vi "Editor_UI_Main.vi"(11 "manager_daemon":refnum<class "manager_daemon.lvclass">) -> ()   [LabVIEW 2024]
uses:
  <vilib>/sklein/WebView2/Webview2 Control/WebView2 Control.xctl
  CV_Shared_Library/volume.type--enum.ctl
  comic_manager/manager_daemon/manager_daemon.lvclass
  comic_manager/manager_daemon/manager_daemon.lvclass/manager_daemon.ctl
  <vilib>/addons/_JKI Toolkits/State Machine/_JKI_lib_State_Machine.llb/Select State(s)_err__jki_lib_state_machine.vi
  <vilib>/addons/_JKI Toolkits/State Machine/_JKI_lib_State_Machine.llb/Periodic Trigger__ogtk__JKI-SM__jki_lib_state_machine.vi
  <userlib>/_OpenG.lib/file/file.llb/Strip Path Extension - String__ogtk.vi
  <userlib>/_OpenG.lib/file/file.llb/openg_file.lvlib
  <vilib>/addons/_JKI.lib/Serialization/JSON/JKI JSON Serialization.lvlib
  CV_Shared_Library/CV_Shared_Library.lvlib
  <userlib>/_OpenG.lib/array/array.llb/openg_array.lvlib
  comic_manager/manager_daemon/type_defs/VolumeData--cluster.ctl
  comic_manager/manager_daemon/type_defs/IssueData--clustrer.ctl
  <userlib>/_OpenG.lib/array/array.llb/Remove Duplicates from 1D Array (Variant)__ogtk.vi
panel:
  out "target volume":string
  in  "delete issue":bool caption="delete current"
  in  "use rel date":bool caption="delete current"
  out "issue chart":picture
  in  "fix dates":bool caption="delete current"
  out "dup issue dates":string[](array[string])
  out "Unique Dates":bool
  in  "delete volume":bool caption="delete current"
  out "URL":string
  in  "refresh listings":bool
  in  "commit volume type":bool
  in  "volume type":T1 caption="Enum"
  out "last updated":string
  in  "Volume":i32 caption="Numeric"
  in  "issue detail tab control":enum32{"Details", "Cover", "Lists"}(tab)
  out "Rel Date":timestamp format="%<%x>T"
  out "Issue ID":i32 caption="Numeric"
  out "Issue Title":string
  in  "Cover Date":timestamp format="%<%x>T"
  out "Issue Number":string
  in  "issue description":string(xcontrol)
  in  "issue cover":string(xcontrol)
  out "Characters":string[](array[string])
  out "Teams":string[](array[string])
  out "StoryArcs":string[](array[string])
  out "Creators":string[](array[string])
  out "Concepts":string[](array[string])
  in  "sort volume":bool
  in  "to top":bool
  in  "move down":bool
  in  "move up":bool
  in  "issues":i32(listbox)
  out "Start Year":i32 caption="Numeric"
  out "issue count":i32 caption="Numeric"
  out "Sortable Title":string
  in  "Title":string
  in  "volume description":string(xcontrol)
  in  "volumes":i32(listbox)
  in  "Folder":i32(listbox)
  in  "Exit":bool
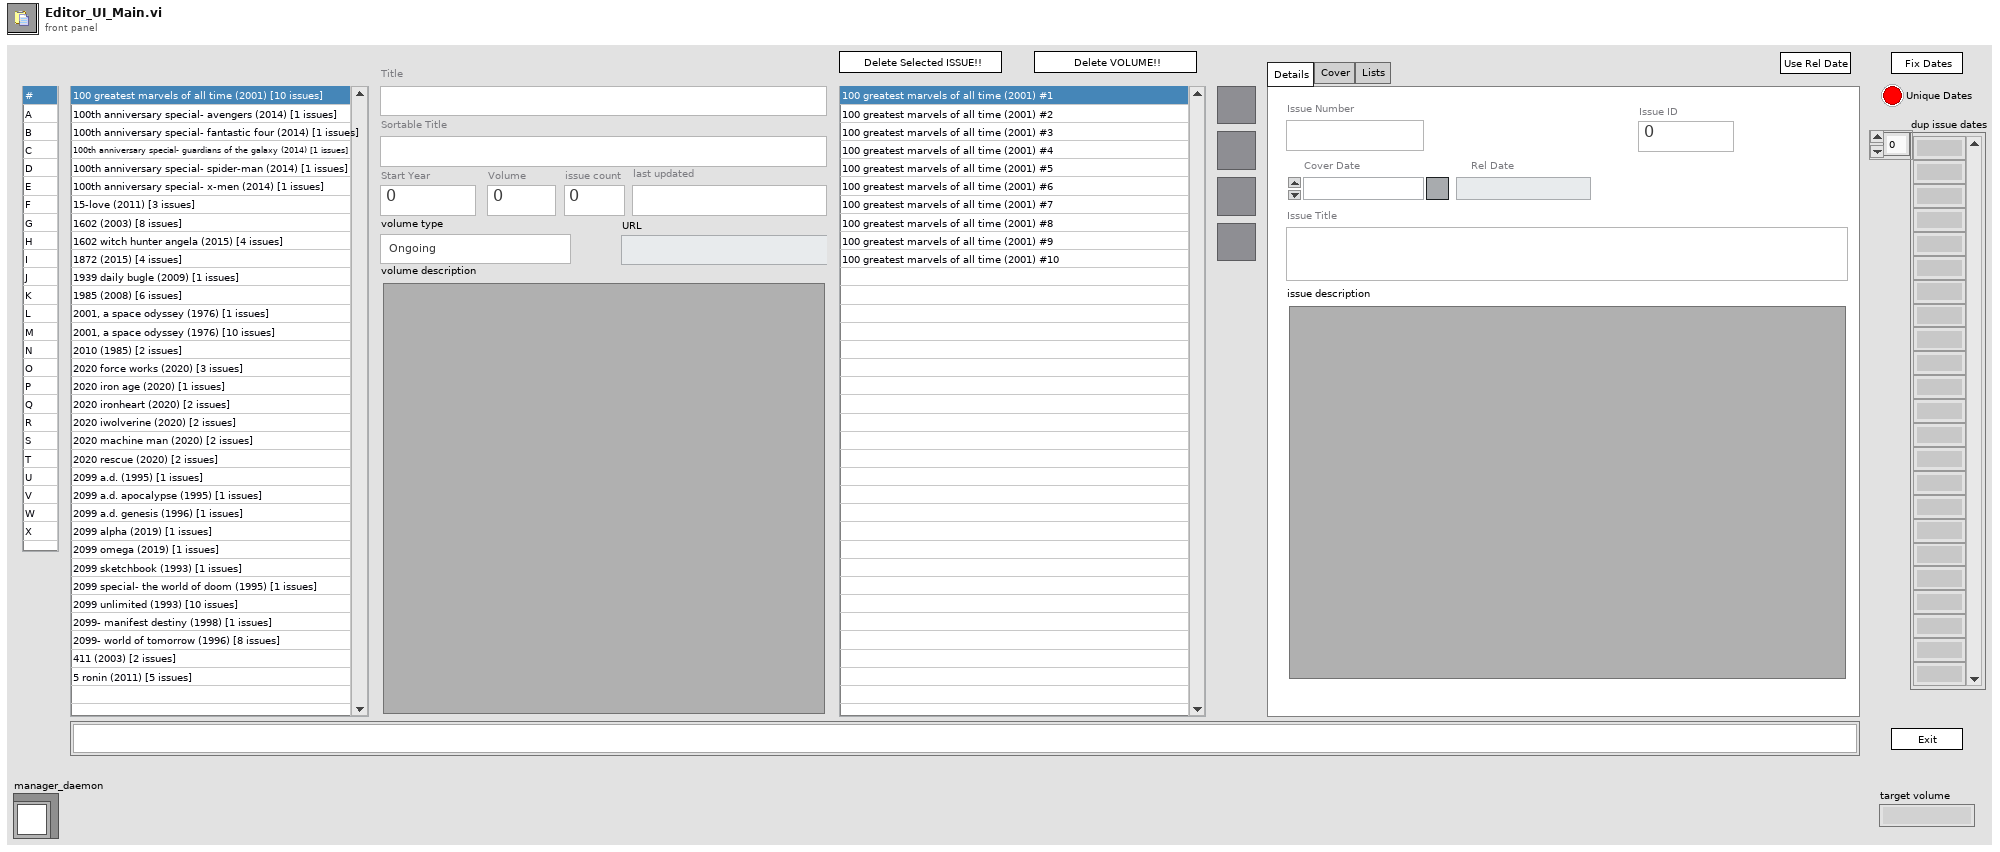
[diagram p1: front panel]
types:
  T1 = typedef "CV_Shared_Library.lvlib/volume.type--enum.ctl" = enum16{"Ongoing", "Limited Series", "Annual", "One Shot", "Reprint/Document", "Star Comics", "Epic Comics"}
  T2 = enum32{"Invalid", "Standard", "Closed", "Hidden", "Minimized", "Maximized"}
  T3 = enum32{"invalid app kind", "Development System", "Run Time System", "Student Edition", "Embedded LabVIEW", "Evaluation", "Custom"}
  T4 = typedef "manager_daemon.lvclass/VolumeData--cluster.ctl" = cluster{"name":string, "sortable_name":string, "aliases":string[], "description":string, "site_detail_url":string, "count_of_issues":i32, "start_year":i32, "publisher_id":i32, "issue_ids":i32[], "date_last_updated":timestamp, "volume":i32, "cv_id":string, "volume type":T1, "source_path":path}
  T5 = typedef "manager_daemon.lvclass/IssueData--clustrer.ctl" = cluster{"cover_date":timestamp, "cv_id":string, "name":string, "sortable_name":string, "issue_number":string, "deck":string, "description":string, "id":i32, "store_date":timestamp, "date_last_updated":timestamp, "site_detail_url":string, "cover_url":string, "source_path":path}
  T6 = cluster{"Core":cluster{"Current VI Reference":refnum<vi>, "Close Panel on Exit?":bool}, "cv_vols":path[], "vol  filter map":map{i32, map{string, i32}}, "current volume map":map{string, i32}, "volume":T4, "issues":T5[], "root paths":cluster{"cv_volumes":path, "cv_issues":path}, "dup issues":i32[], "manager_daemon":refnum<class "manager_daemon.lvclass">, "new volume":string, "Refresh all":bool}
  T7 = cluster{"Current VI Reference":refnum<vi>, "Close Panel on Exit?":bool}
  T8 = typedef "WebView2 Control.xctl/Events.ctl" = cluster{"Navigation Complete Event":refnum<user-event>, "Source Changed Event":refnum<user-event>, "Document Title Changed Event":refnum<user-event>, "Status Bar Text Changed":refnum<user-event>, "Web Message Received":refnum<user-event>, "Window Close Requested":refnum<user-event>, "DOM Loaded":refnum<user-event>, "Navigation Started Event":refnum<user-event>}
  T9 = typedef "CV_RESTful_Lib.lvlib/local_issue--cluster.ctl" = cluster{"cover_date":timestamp, "id":i32, "cv_id":string, "name":string, "sortable_name":string, "issue_number":string, "deck":string, "description":string, "volume":T10, "store_date":timestamp, "date_last_updated":timestamp, "site_detail_url":string, "cover_url":string, "associated_images":T11[], "characters":T10[], "concepts":T10[], "creators":T12[], "storyArcs":T10[], "teams":T10[]}
  T10 = typedef "CV_RESTful_Lib.lvlib/cv_issue.generic_credit--cluster.ctl" = cluster{"id":i32, "name":string}
  T11 = typedef "CV_RESTful_Lib.lvlib/cv_issue.associated_image--cluster.ctl" = cluster{"original_url":string, "id":i32}
  T12 = typedef "CV_RESTful_Lib.lvlib/cv_issue.person_credit--cluster.ctl" = cluster{"id":i32, "name":string, "role":string}
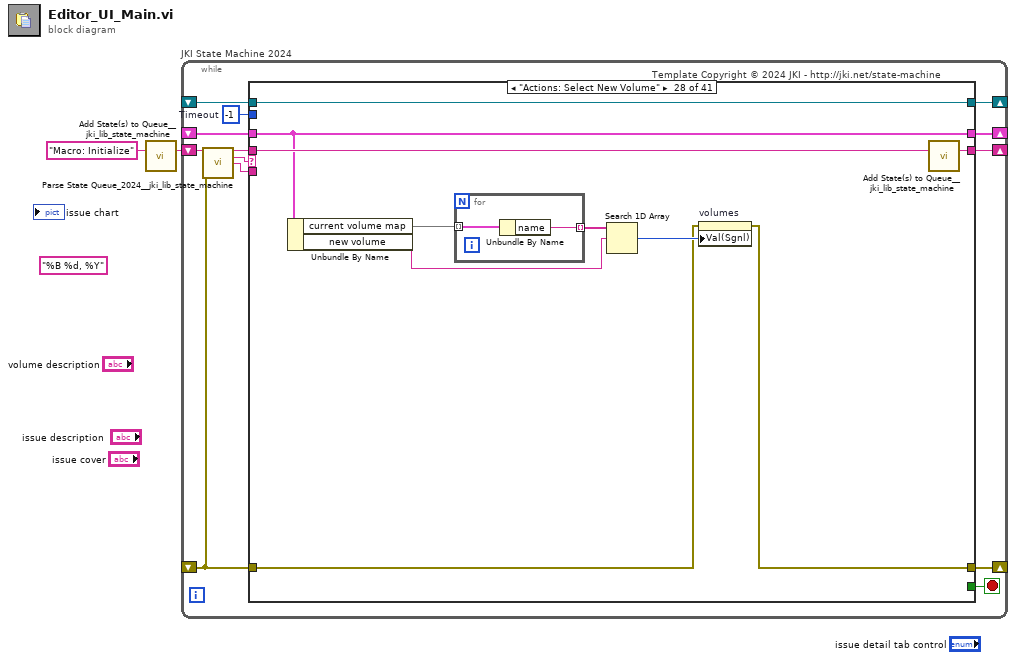
[diagram p0: block diagram]
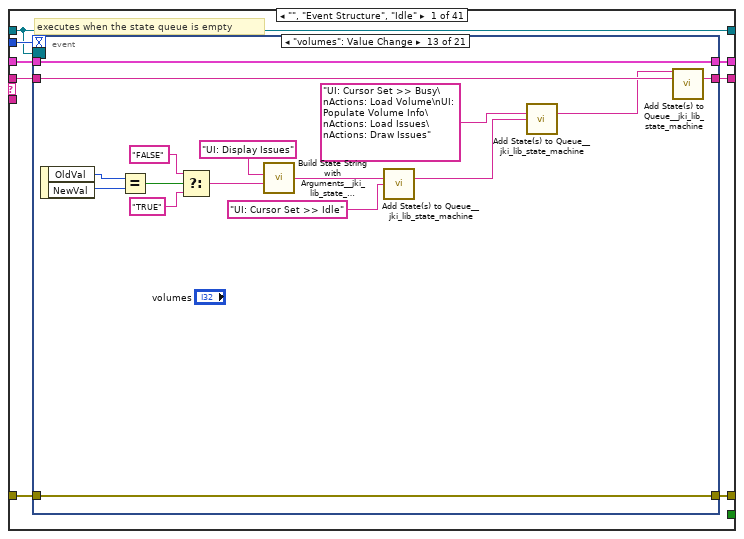
[diagram p2: hidden frame]
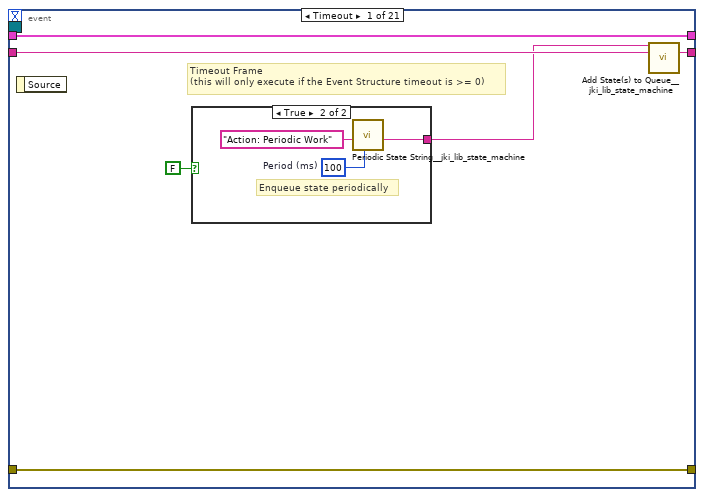
[diagram p3: hidden frame]
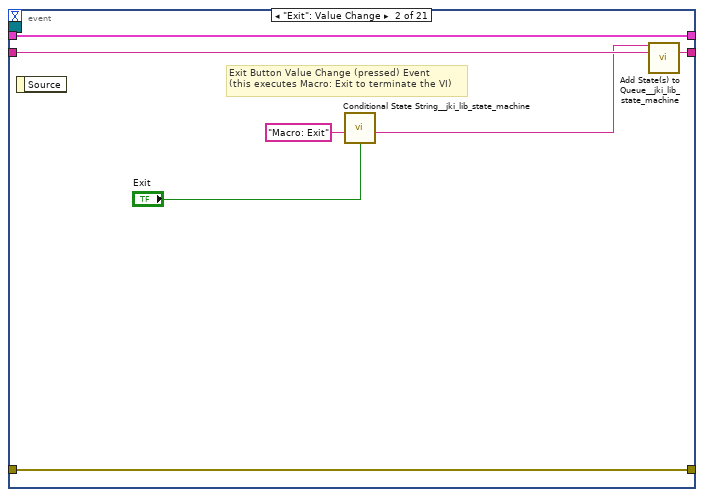
[diagram p5: hidden frame]
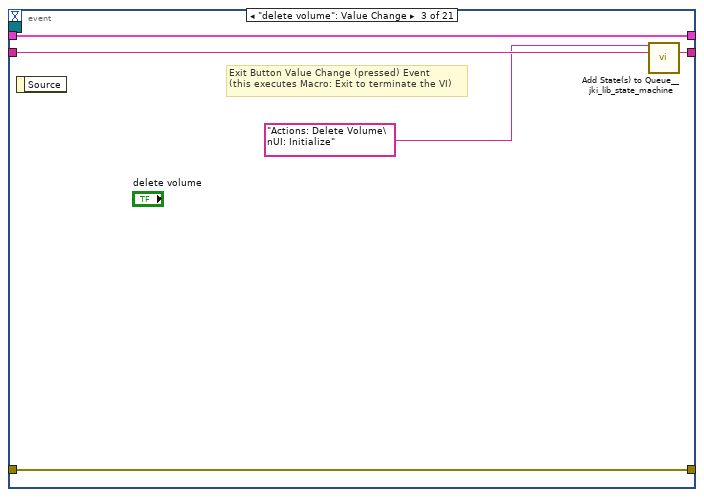
[diagram p6: hidden frame]
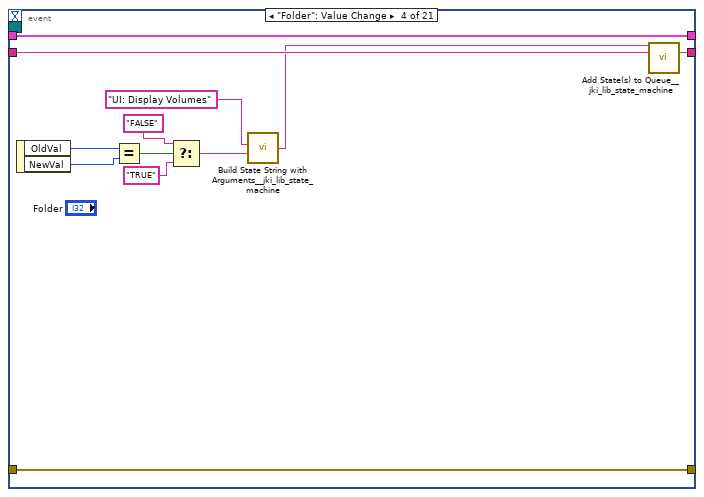
[diagram p7: hidden frame]
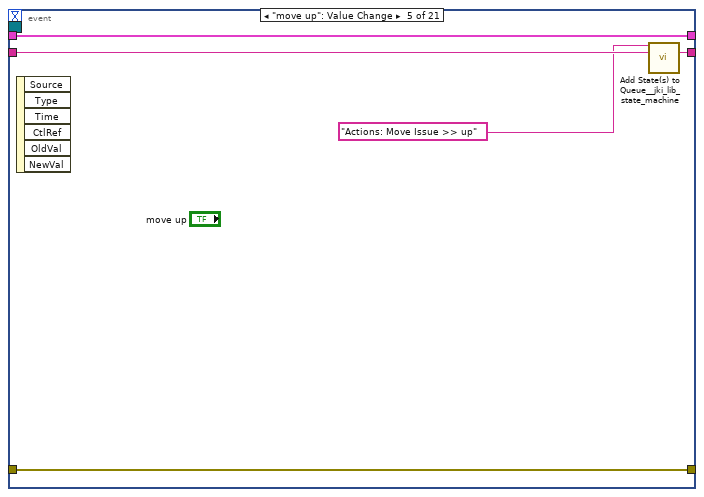
[diagram p8: hidden frame]
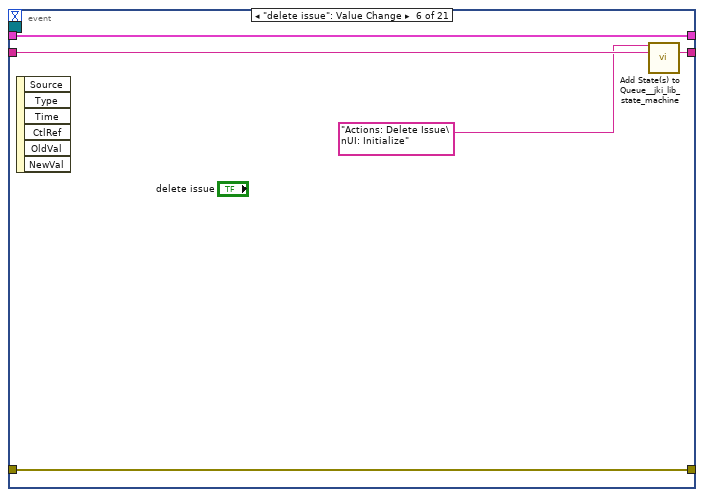
[diagram p9: hidden frame]
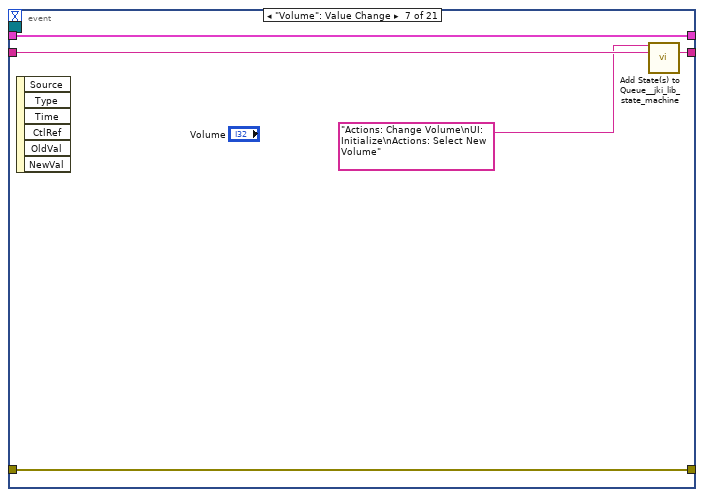
[diagram p10: hidden frame]
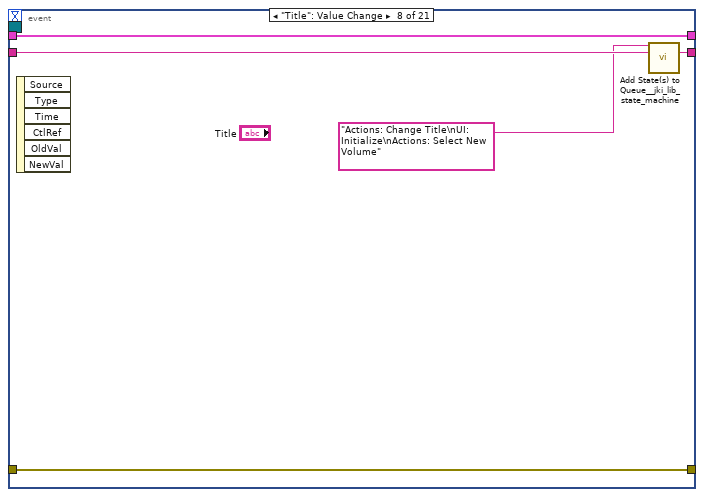
[diagram p11: hidden frame]
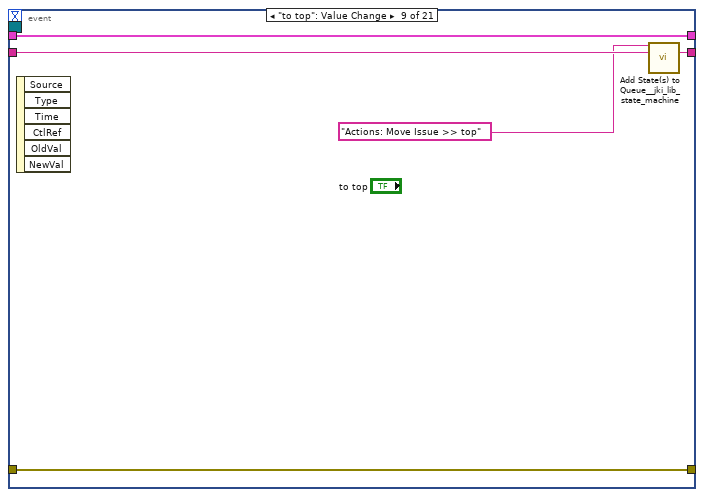
[diagram p12: hidden frame]
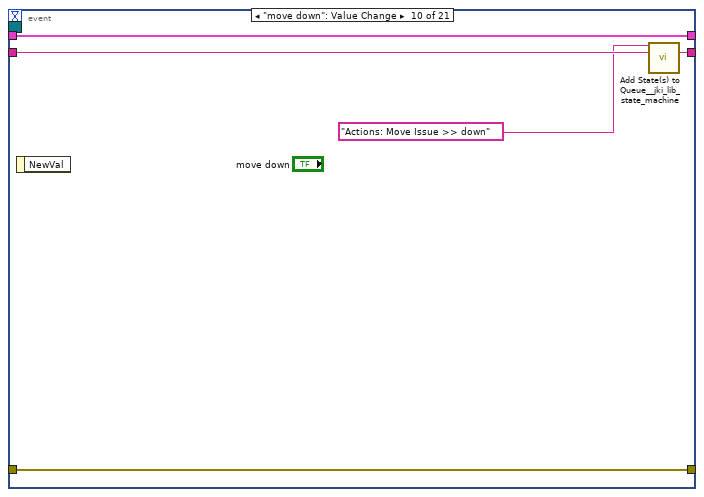
[diagram p13: hidden frame]
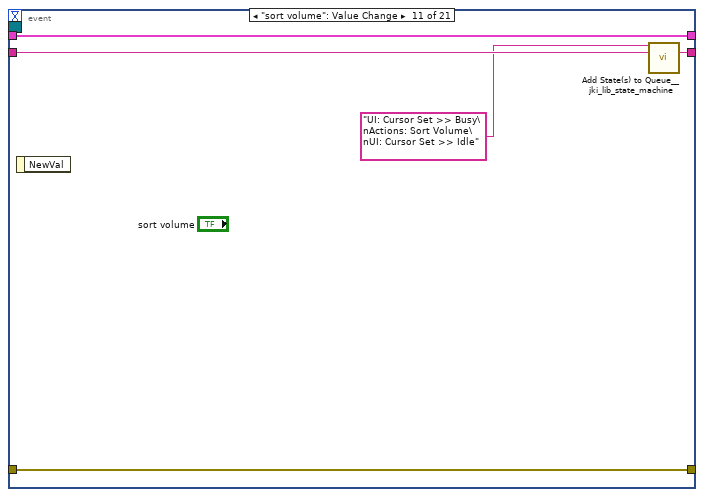
[diagram p14: hidden frame]
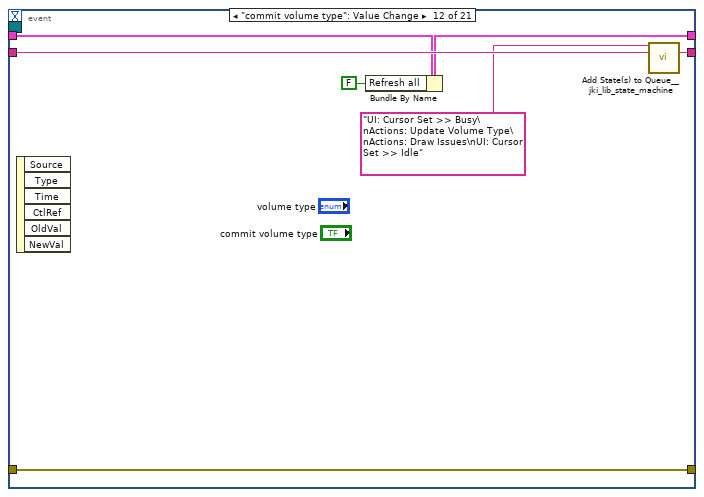
[diagram p15: hidden frame]
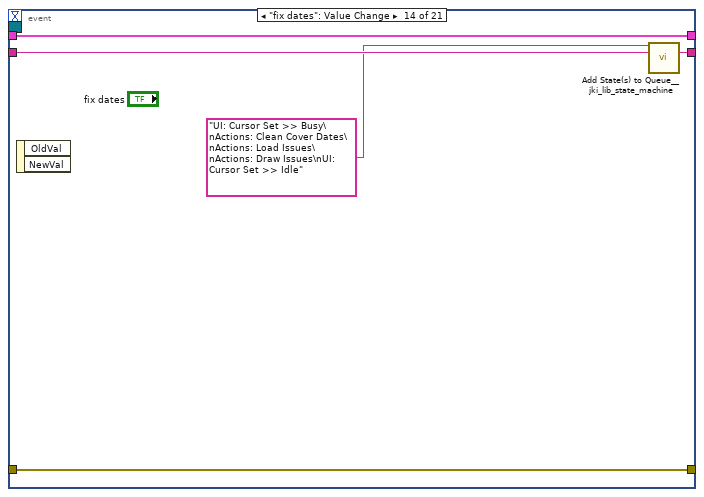
[diagram p16: hidden frame]
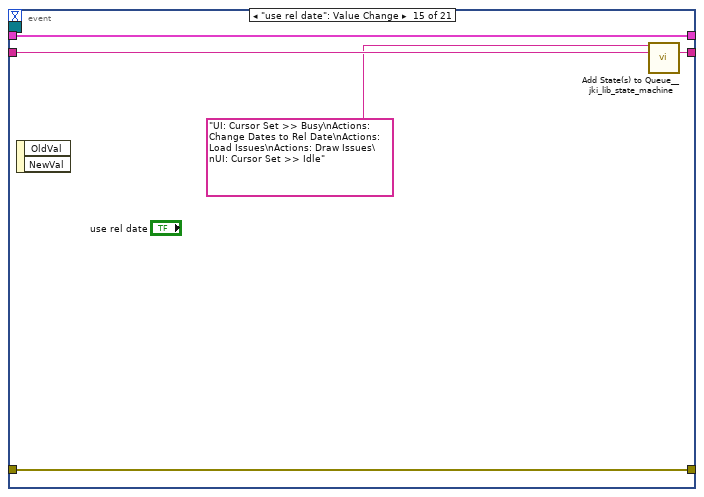
[diagram p17: hidden frame]
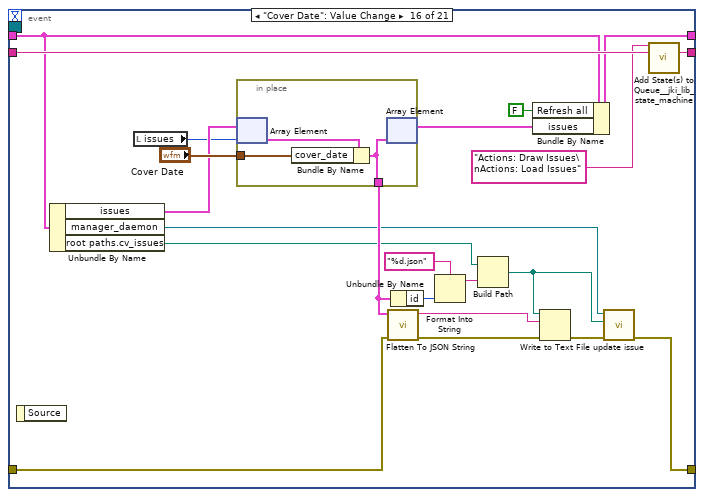
[diagram p18: hidden frame]
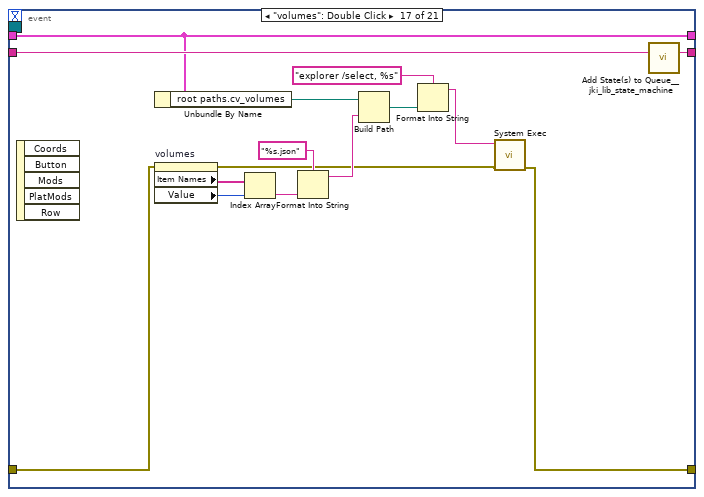
[diagram p19: hidden frame]
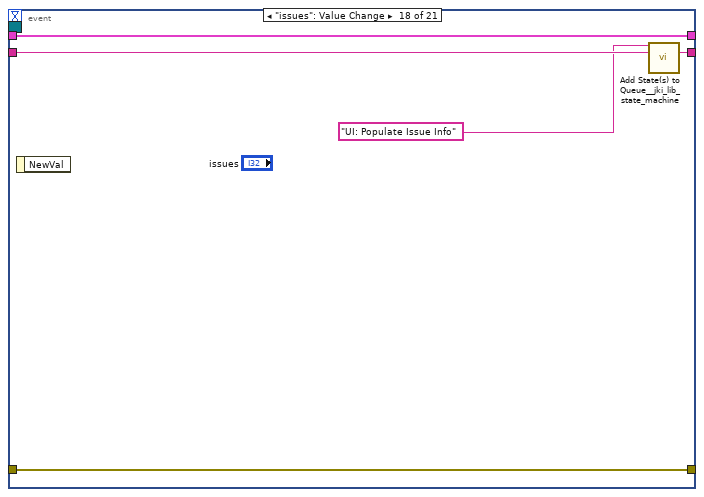
[diagram p20: hidden frame]
diagram:
  (unwired) "%B %d, %Y" ("time format string (%c)")
  n1 = call <vilib>:"Add State(s) to Queue__jki_lib_state_machine.vi"("State(s) in (\"\")"="Macro: Initialize") -> ("States Out"=w2:string)  [unwired: 14 in]
  n2 = while "JKI State Machine 2024" {
    shift-right: [w8] -> _
    shift-left: _ -> [w7]
    shift-right: [w11] -> _
    shift-left: _ -> [w5]
    shift-right: [w10] -> _
    shift-left: w2 -> [w12]
    shift-right: [w4] -> _
    shift-left: _ -> [w3]
    stop <- w9 stop-if-true
    w6 = -1  # Timeout
    # "Template Copyright © 2024 JKI - http://jki.net/state-machine"
    n3 = call <vilib>:"Parse State Queue_2024__jki_lib_state_machine.vi"("State Queue"=w12, "Error In (no error)"=w5) -> ("Remaining States"=w14:string, "Current State"=w15:string, "Arguments"=w13:string)  [unwired: 11 in]
    n4 = case shown="\"Actions: Select New Volume\"" w15 {
      selector: w15 -> [_ _ w217 _ _ _ _ _ _ _ _ _ _ _ _ _ _ _ _ _ _ _ _ _ _ _ _ _ _ _ _ _ _ _ _ _ _ _ _ _ _]
      tunnel: w14 -> [w23 w215 w221 w241 w252 w262 w267 w283 w290 w295 w308 w314 w319 w334 w364 w385 w401 w430 w449 w454 w461 w473 w543 w549 w559 w564 w587 w597 w627 w640 w665 w682 w712 w734 w747 w771 w797 w811 w830 w846 w854]
      tunnel: w13 -> [_ _ _ _ w247 _ _ _ _ _ _ _ _ w322 w356 _ _ _ _ _ w456 w467 _ _ _ _ _ _ _ _ _ _ _ _ _ w753 _ _ _ _ _]
      tunnel: w7 -> [w21 w212 w219 w234 w249 w260 w264 _ w285 w292 w299 w312 w316 w330 w359 w382 w396 w427 w447 w452 w459 w469 w540 w546 w557 w561 w583 w594 w622 w635 w662 w677 w709 w730 w744 w750 w786 w808 w828 w838 w850]
      tunnel: [w20 w213 w223 w238 errorcluster {"status"=FALSE, "code"=0, "source"=""} ("error out") w259 w265 w280 w286 w293 w301 w309 w317 w325 w360 w383 w398 w416 w446 w451 w457 w470 w541 w547 w554 w562 w573 w588 w604 w630 w656 w671 w697 w723 w742 w760 w792 w800 w812 w841 w848] -> w11
      tunnel: w5 -> [w17 w213 w222 w238 w248 w259 w265 w280 w287 w293 w303 w310 w317 w326 w361 w383 w399 w419 w446 w451 w458 w471 w541 w547 w554 w562 w579 w589 w617 w632 w657 w673 w703 w731 w738 w752 w783 w801 w816 w840 w852]
      tunnel: [w22 w214 w220 w240 w251 w261 w266 w282 w289 w294 w307 w313 w318 w333 w363 w384 w400 w429 w448 w453 w460 w472 w542 w548 w558 w563 w586 w596 w626 w639 w664 w681 w711 w733 w746 w770 w796 w810 w830 w845 w854] -> w10
      tunnel: [_ _ _ _ _ TRUE _ _ _ _ _ _ _ _ _ _ _ _ _ _ _ _ _ _ _ _ _ _ _ _ _ _ _ _ _ _ _ _ _ _ _] -> w9
      tunnel: [w19 w212 w219 w239 w249 w260 w264 w281 w285 w292 w299 w312 w316 w329 w359 w382 w396 w427 w447 w452 w459 w469 w540 w546 w557 w561 w584 w594 w624 w633 w662 w676 w709 w730 w737 w749 w785 w807 w827 w842 w853] -> w8
      tunnel: w6 -> [w18 _ _ _ _ _ _ _ _ _ _ _ _ _ _ _ _ _ _ _ _ _ _ _ _ _ _ _ _ _ _ _ _ _ _ _ _ _ _ _ _]
      tunnel: [w16 w211 w216 w228 w242 w257 w263 w277 w284 w291 w304 w311 w315 w324 w362 w381 w397 w428 w444 w450 w455 w466 w539 w544 w550 w560 w585 w595 w625 w638 w663 w680 w710 w732 w745 w769 w795 w809 w829 w839 w851] -> w4
      tunnel: w3 -> [w16 w211 w216 w228 w242 w257 w263 w277 w284 w291 _ w311 w315 w324 w362 w381 w397 w428 w444 w450 w455 w466 w539 w544 w550 w560 w585 w595 w625 w638 w663 w680 w710 w732 w745 w769 w795 w809 w829 w839 w851]
      frame "", "Event Structure", "Idle" {
        # "executes when the state queue is empty"
        n5 = event shown="[12] \"volumes\": Value Change" {
          selector: w16 -> [_ _ _ _ _ _ _ _ _ _ _ _ _ _ _ _ _ _ _ _ _]
          dyn-events: _ -> [_ _ _ _ _ _ _ _ _ _ _ _ _ _ _ _ _ _ _ _ _]
          timeout: w18 -> [_ _ _ _ _ _ _ _ _ _ _ _ _ _ _ _ _ _ _ _ _]
          tunnel: w23 -> [w29 w39 w44 w56 w61 w66 w71 w76 w81 w86 w91 w98 w114 w119 w124 w146 w164 w169 w180 w192 w210]
          tunnel: [w28 w38 w43 w55 w60 w65 w70 w75 w80 w85 w90 w97 w113 w118 w123 w145 w163 w168 w179 w192 w209] -> w22
          tunnel: w21 -> [w26 w36 w41 w53 w58 w63 w68 w73 w78 w83 w88 w94 w111 w116 w121 w141 w158 w166 w174 w193 w207]
          tunnel: [w27 w37 w42 w54 w59 w64 w69 w74 w79 w84 w89 w96 w112 w117 w122 w129 w150 w167 w178 w188 w208] -> w20
          tunnel: w17 -> [w27 w37 w42 w54 w59 w64 w69 w74 w79 w84 w89 w96 w112 w117 w122 w138 w155 w167 w178 w203 w208]
          tunnel: [w26 w36 w41 w53 w58 w63 w68 w73 w78 w83 w88 w93 w111 w116 w121 w139 w158 w166 w170 w193 w207] -> w19
          event Timeout {
            # "Timeout Frame\n(this will only execute if the Event Structure timeout is >= 0)"
            n6 = event-data() -> ()  [unwired: 1 in, 1 out]
            n7 = case shown="True" FALSE {
              tunnel: [_ w32] -> w25
              frame False {
              }
              frame True {
                w30 = u32 100  # Period (ms)
                # "Enqueue state periodically"
                n8 = call <vilib>:"Periodic State String__jki_lib_state_machine.vi"("Period (ms)"=w30, "State"="Action: Periodic Work") -> ("State Out"=w32:string)  [unwired: 9 in]
              }
            }
            n9 = call <vilib>:"Add State(s) to Queue__jki_lib_state_machine.vi"("State(s) in Front (\"\")"=w25, "State(s) in (\"\")"=w29) -> ("States Out"=w28:string)  [unwired: 13 in]
          }
          event "Exit": Value Change {
            # "Exit Button Value Change (pressed) Event\n(this executes Macro: Exit to terminate the VI)"
            n10 = event-data() -> ()  [unwired: 1 in, 1 out]
            n11 = call <vilib>:"Conditional State String__jki_lib_state_machine.vi"("Do State(s)?"="Exit", "State"="Macro: Exit") -> ("State Out"=w33:string)  [unwired: 7 in]
            n12 = call <vilib>:"Add State(s) to Queue__jki_lib_state_machine.vi"("State(s) in Front (\"\")"=w33, "State(s) in (\"\")"=w39) -> ("States Out"=w38:string)  [unwired: 13 in]
          }
          event "delete volume": Value Change {
            # "Exit Button Value Change (pressed) Event\n(this executes Macro: Exit to terminate the VI)"
            n13 = event-data() -> ()  [unwired: 1 in, 1 out]
            n14 = call <vilib>:"Add State(s) to Queue__jki_lib_state_machine.vi"("State(s) in Front (\"\")"="Actions: Delete Volume\nUI: Initialize", "State(s) in (\"\")"=w44) -> ("States Out"=w43:string)  [unwired: 13 in]
          }
          event "Folder": Value Change {
            n15 = event-data() -> ("OldVal"=w52:i32, "NewVal"=w51:i32)  [unwired: 1 in]
            n16 = Equal?(x=w52, y=w51) -> (x = y?=w50:bool)
            n17 = Select(t="FALSE", s=w50, f="TRUE") -> (s? t:f=w46:string)
            n18 = call <vilib>:"Build State String with Arguments__jki_lib_state_machine.vi"("Arguments (\"\")"=w46, "State"="UI: Display Volumes") -> ("State with Arguments"=w45:string)  [unwired: 4 in]
            n19 = call <vilib>:"Add State(s) to Queue__jki_lib_state_machine.vi"("State(s) in Front (\"\")"=w45, "State(s) in (\"\")"=w56) -> ("States Out"=w55:string)  [unwired: 13 in]
          }
          event "move up": Value Change {
            n20 = event-data() -> ()  [unwired: 1 in, 6 out]
            n21 = call <vilib>:"Add State(s) to Queue__jki_lib_state_machine.vi"("State(s) in Front (\"\")"="Actions: Move Issue >> up", "State(s) in (\"\")"=w61) -> ("States Out"=w60:string)  [unwired: 13 in]
          }
          event "delete issue": Value Change {
            n22 = event-data() -> ()  [unwired: 1 in, 6 out]
            n23 = call <vilib>:"Add State(s) to Queue__jki_lib_state_machine.vi"("State(s) in Front (\"\")"="Actions: Delete Issue\nUI: Initialize", "State(s) in (\"\")"=w66) -> ("States Out"=w65:string)  [unwired: 13 in]
          }
          event "Volume": Value Change {
            n24 = event-data() -> ()  [unwired: 1 in, 6 out]
            n25 = call <vilib>:"Add State(s) to Queue__jki_lib_state_machine.vi"("State(s) in Front (\"\")"="Actions: Change Volume\nUI: Initialize\nActions: Select New Volume", "State(s) in (\"\")"=w71) -> ("States Out"=w70:string)  [unwired: 13 in]
          }
          event "Title": Value Change {
            n26 = event-data() -> ()  [unwired: 1 in, 6 out]
            n27 = call <vilib>:"Add State(s) to Queue__jki_lib_state_machine.vi"("State(s) in Front (\"\")"="Actions: Change Title\nUI: Initialize\nActions: Select New Volume", "State(s) in (\"\")"=w76) -> ("States Out"=w75:string)  [unwired: 13 in]
          }
          event "to top": Value Change {
            n28 = event-data() -> ()  [unwired: 1 in, 6 out]
            n29 = call <vilib>:"Add State(s) to Queue__jki_lib_state_machine.vi"("State(s) in Front (\"\")"="Actions: Move Issue >> top", "State(s) in (\"\")"=w81) -> ("States Out"=w80:string)  [unwired: 13 in]
          }
          event "move down": Value Change {
            n30 = event-data() -> ()  [unwired: 1 in, 1 out]
            n31 = call <vilib>:"Add State(s) to Queue__jki_lib_state_machine.vi"("State(s) in Front (\"\")"="Actions: Move Issue >> down", "State(s) in (\"\")"=w86) -> ("States Out"=w85:string)  [unwired: 13 in]
          }
          event "sort volume": Value Change {
            n32 = event-data() -> ()  [unwired: 1 in, 1 out]
            n33 = call <vilib>:"Add State(s) to Queue__jki_lib_state_machine.vi"("State(s) in Front (\"\")"="UI: Cursor Set >> Busy\nActions: Sort Volume\nUI: Cursor Set >> Idle", "State(s) in (\"\")"=w91) -> ("States Out"=w90:string)  [unwired: 13 in]
          }
          event "commit volume type": Value Change {
            n34 = event-data() -> ()  [unwired: 1 in, 6 out]
            n35 = Bundle By Name(cluster=w94, "Refresh all"=FALSE) -> (w93:T6)
            n36 = call <vilib>:"Add State(s) to Queue__jki_lib_state_machine.vi"("State(s) in Front (\"\")"="UI: Cursor Set >> Busy\nActions: Update Volume Type\nActions: Draw Issues\nUI: Cursor Set >> Idle", "State(s) in (\"\")"=w98) -> ("States Out"=w97:string)  [unwired: 13 in]
          }
          event "volumes": Value Change {
            n37 = event-data() -> ("OldVal"=w109:i32, "NewVal"=w110:i32)  [unwired: 1 in]
            n38 = Equal?(x=w109, y=w110) -> (x = y?=w106:bool)
            n39 = Select(t="FALSE", s=w106, f="TRUE") -> (s? t:f=w104:string)
            n40 = call <vilib>:"Build State String with Arguments__jki_lib_state_machine.vi"("Arguments (\"\")"=w104, "State"="UI: Display Issues") -> ("State with Arguments"=w101:string)  [unwired: 4 in]
            n41 = call <vilib>:"Add State(s) to Queue__jki_lib_state_machine.vi"("State(s) in (\"\")"=w101, "State(s) at Back (\"\")"="UI: Cursor Set >> Idle" ("State(s) at Back (\"\")")) -> ("States Out"=w100:string)  [unwired: 13 in]
            n42 = call <vilib>:"Add State(s) to Queue__jki_lib_state_machine.vi"("State(s) in (\"\")"="UI: Cursor Set >> Busy\nActions: Load Volume\nUI: Populate Volume Info\nActions: Load Issues\nActions: Draw Issues", "State(s) at Back (\"\")"=w100) -> ("States Out"=w107:string)  [unwired: 13 in]
            n43 = call <vilib>:"Add State(s) to Queue__jki_lib_state_machine.vi"("State(s) in Front (\"\")"=w107, "State(s) in (\"\")"=w114) -> ("States Out"=w113:string)  [unwired: 13 in]
          }
          event "fix dates": Value Change {
            n44 = event-data() -> ()  [unwired: 1 in, 2 out]
            n45 = call <vilib>:"Add State(s) to Queue__jki_lib_state_machine.vi"("State(s) in Front (\"\")"="UI: Cursor Set >> Busy\nActions: Clean Cover Dates\nActions: Load Issues\nActions: Draw Issues\nUI: Cursor Set >> Idle", "State(s) in (\"\")"=w119) -> ("States Out"=w118:string)  [unwired: 13 in]
          }
          event "use rel date": Value Change {
            n46 = event-data() -> ()  [unwired: 1 in, 2 out]
            n47 = call <vilib>:"Add State(s) to Queue__jki_lib_state_machine.vi"("State(s) in Front (\"\")"="UI: Cursor Set >> Busy\nActions: Change Dates to Rel Date\nActions: Load Issues\nActions: Draw Issues\nUI: Cursor Set >> Idle", "State(s) in (\"\")"=w124) -> ("States Out"=w123:string)  [unwired: 13 in]
          }
          event "Cover Date": Value Change {
            n48 = event-data() -> ()  [unwired: 1 in, 1 out]
            n49 = Unbundle By Name(w141) -> ("issues"=w143:T5[], "manager_daemon"=w127:refnum<class "manager_daemon.lvclass">, "root paths.cv_issues"=w128:path)
            n50 = local read "issues"() -> (w142:i32)
            n51 = in-place {
              in-place-border: "Cover Date" -> [w148]
              in-place-border: [w147] -> w137
              n52 = in-place-array #1(w143, w142) -> (w149:T5)
              n53 = Bundle By Name(cluster=w149, "cover_date"=w148) -> (w147:T5)
              n54 = in-place-array #1(w147) -> (w140:T5[])  [unwired: 1 out]
            }
            n55 = call <vilib>:"Flatten To JSON String.vi"("error in"=w138, "Variant"=w137) -> ("error out"=w132:errorcluster, "JSON String"=w133:string)  [unwired: 8 in]
            n56 = Unbundle By Name(w137) -> ("id"=w136:i32)
            n57 = Format Into String(format string="%d.json", w136) -> (resulting string=w134:string)  [unwired: 2 in, 1 out]
            n58 = Build Path(base path=w128, name or relative path=w134) -> (appended path=w126:path)
            n59 = Bundle By Name(cluster=w141, "Refresh all"=FALSE, "issues"=w140) -> (w139:T6)
            n60 = Write to Text File(file (use dialog)=w126, text=w133, error in=w132) -> (error out=w130:errorcluster)  [unwired: 1 in, 2 out]
            n61 = call "update issue.vi"("error in (no error)"=w130, "Issue Path"=w126, "manager_daemon in"=w127) -> ("error out"=w129:errorcluster)  [unwired: 7 in, 1 out]
            n62 = call <vilib>:"Add State(s) to Queue__jki_lib_state_machine.vi"("State(s) in Front (\"\")"="Actions: Draw Issues\nActions: Load Issues" ("State(s) in Front (\"\")"), "State(s) in (\"\")"=w146) -> ("States Out"=w145:string)  [unwired: 13 in]
          }
          event "volumes": Double Click {
            n63 = event-data() -> ()  [unwired: 1 in, 5 out]
            n64 = Unbundle By Name(w158) -> ("root paths.cv_volumes"=w157:path)
            n65 = property on="volumes" class="LstBox (strict)"(error in=w155) -> (error out=w151:errorcluster, "Item Names"=w161:string[], "Value"=w162:i32)  [unwired: 1 in, 1 out]
            n66 = Index Array(array=w161, index=w162) -> (element=w159:string)
            n67 = Format Into String(format string="%s.json", w159) -> (resulting string=w156:string)  [unwired: 2 in, 1 out]
            n68 = Build Path(base path=w157, name or relative path=w156) -> (appended path=w153:path)
            n69 = Format Into String(format string="explorer /select, %s", w153) -> (resulting string=w152:string)  [unwired: 2 in, 1 out]
            n70 = call <vilib>:"System Exec.vi"("error in (no error)"=w151, "command line"=w152) -> ("error out"=w150:errorcluster)  [unwired: 6 in, 3 out]
            n71 = call <vilib>:"Add State(s) to Queue__jki_lib_state_machine.vi"("State(s) in (\"\")"=w164) -> ("States Out"=w163:string)  [unwired: 14 in]
          }
          event "issues": Value Change {
            n72 = event-data() -> ()  [unwired: 1 in, 1 out]
            n73 = call <vilib>:"Add State(s) to Queue__jki_lib_state_machine.vi"("State(s) in Front (\"\")"="UI: Populate Issue Info", "State(s) in (\"\")"=w169) -> ("States Out"=w168:string)  [unwired: 13 in]
          }
          event "refresh listings": Value Change; User Event {
            (unwired) "UI: Initialize\nActions: Select New Volume"
            n74 = event-data() -> ()  [unwired: 1 in, 3 out]
            n75 = property on="volumes" class="LstBox (strict)"() -> ("Item Names"=w176:string[], "Value"=w175:i32)  [unwired: 2 in, 2 out]
            n76 = Unbundle By Name(w174) -> ("Refresh all"=w173:bool)
            n77 = case shown="True" w173 {
              tunnel: [_ "UI: Initialize"] -> w177
              tunnel: w176 -> [_ w186]
              tunnel: w175 -> [_ w185]
              tunnel: w174 -> [w181 w184]
              tunnel: [w181 w182] -> w172
              frame False {
              }
              frame True {
                n78 = Index Array(array=w186, index=w185) -> (element=w183:string)
                n79 = Bundle By Name(cluster=w184, "new volume"=w183) -> (w182:T6)
              }
            }
            n80 = Bundle By Name(cluster=w172, "Refresh all"=TRUE) -> (w170:T6)
            n81 = call <vilib>:"Add State(s) to Queue__jki_lib_state_machine.vi"("State(s) in Front (\"\")"=w177, "State(s) in (\"\")"=w180) -> ("States Out"=w179:string)  [unwired: 13 in]
          }
          event User Event {
            n82 = event-data() -> ("display volume"=w194:string)  [unwired: 1 in]
            "target volume" <- w194
            n83 = property on="Folder" class="LstBox (strict)"(error in=w203) -> (error out=w195:errorcluster, "Item Names"=w202:string[])  [unwired: 1 in, 1 out]
            n84 = String Subset(string=w194, length (rest)=1 ("length (rest)")) -> (substring=w200:string)  [unwired: 1 in]
            n85 = To Lower Case(string=w202) -> (all lower case string=w201:string[])
            n86 = Search 1D Array(1D array=w201, element=w200) -> (index of element=w198:i32)  [unwired: 1 in]
            n87 = Less Than 0?(x=w198) -> (x < 0?=w199:bool)
            n88 = Select(t=0, s=w199, f=w198) -> (s? t:f=w196:i32)
            n89 = property on="Folder" class="LstBox (strict)"(error in=w195, "Val(Sgnl)"=w196) -> (error out=w189:errorcluster)  [unwired: 1 in, 1 out]
            n90 = control-ref of="This VI"() -> (w191:refnum<vi>)
            n91 = property class="VI"(reference=w191, error in=w189, "Front Panel.IsFrontmost"=TRUE ("Front Panel Window:Is Frontmost")) -> (error out=w188:errorcluster)  [unwired: 1 out]
          }
          event Panel Close? {
            # "Discard the event because we'll close the front panel ourselves in Macro: Exit"
            # "Close Panel button (pressed) Event\n(this executes Macro: Exit to terminate the VI)"
            n92 = event-data() -> ()  [unwired: 1 in, 1 out]
            n93 = event-data("Discard?"=TRUE) -> ()  [unwired: 1 in, 1 out]
            n94 = call <vilib>:"Add State(s) to Queue__jki_lib_state_machine.vi"("State(s) in Front (\"\")"="Macro: Exit", "State(s) in (\"\")"=w210) -> ("States Out"=w209:string)  [unwired: 13 in]
          }
        }
      }
      frame "---------- Core ----------" {
        # "Do not put any code in this frame.\n(it is a separator no-op)"
        n95 = call <vilib>:"Add State(s) to Queue__jki_lib_state_machine.vi"("State(s) in (\"\")"=w215) -> ("States Out"=w214:string)  [unwired: 14 in]
      }
      frame Default {
        w226 = 42 items=["No error", "Argument error", "Memory is full", "Out of zone", "End of file", "File already open", "Generic file I/O error", "File not found", "File permission error", "Disk is full", "Duplicate path", "Too many files open", "System feature not enabled", "Resource file not found", "Cannot add resource", "Resource not found", "Image not found", "Image memory error", "Pen does not exist", "Config type invalid", "Config token not found", "Config parse error", "Config memory error", "Bad external code format", "Bad external code offset", "External code not present", "Null window", "Destroy window error", "Null menu", "Print aborted", "Bad print record", "Print driver error", "Windows error during printing", "Memory error during printing", "Print dialog error", "Generic print error", "Invalid device refnum", "Device not found", "Device parameter error", "Device unit error", "Cannot open device", "Device call aborted", "Generic error", "Cancelled by user", "Object ID too low", "Object ID too high", "Object not in heap", "Unknown heap", "Unknown object (invalid DefProc)", "Unknown object (DefProc not in table)", "Message out of range", "Invalid (null) method", "Unknown message", "Manager call not supported", "Bad address", "Network operation in progress", "Network operation timed out", "Connection is busy", "Network attribute not supported", "Network error", "Address in use", "System out of memory", "Connection aborted", "Connection refused", "Not connected", "Already connected", "Connection closed", "Initialization error (interapplication manager)", "Bad occurrence", "Wait on unbound occurrence handler", "Occurrence queue overflow", "Datalog type conflict", "Unused", "Unrecognized type (interapplication manager)", "Memory corrupt", "Failed to make temporary DLL", "Old CIN version", "Drag socket not found", "Failed to load drop-object", "Failed to register OLE object", "Failed to release OLE object", "Format specifier type mismatch", "Unknown format specifier", "Too few format specifiers", "Too many format specifiers", "Scan failed", "Newer CIN version", "Error converting to variant", "Runtime menu error", "Password tampered", "Variant attribute not found", "Incompatible variant data type", "Event data is not available", "Event Store is not present", "Occurrence is not found", "Event Queue is not created", "Event info is not available", "Refnum passed is NULL", "Error retrieving Class GUID", "Error retrieving CoClass GUID", "Error retrieving TypeLib GUID.", "Bad built application magic bytes.", "Specific driver is different from the specific driver associated with the Logical Name.", "There is no session opened to the class driver.", "Max Error", "MAX - Error with config objects", "MAX - Error loading configuration", "MAX - Group not supported"]
        # "Current State"
        # "Do not delete, rename, or modify this frame.\n(this is used to capture unhandled states and typos)"
        # "Handle mistyped state name (developer tool)"
        n96 = Format Into String(format string="Software Exception: Unhandled State \"%s\"." ("message"), error in=w222, w217) -> (resulting string=w225:string, error out=w224:errorcluster)  [unwired: 1 in]
        n97 = call <vilib>:"Error Cluster From Error Code.vi"("show call chain? (False)"=TRUE, "error in (no error)"=w224, "error message (\"\")"=w225, "error code (0)"=w226) -> ("error out"=w223:errorcluster)  [unwired: 5 in]
        n98 = call <vilib>:"Add State(s) to Queue__jki_lib_state_machine.vi"("State(s) in (\"\")"=w221) -> ("States Out"=w220:string)  [unwired: 14 in]
      }
      frame "Initialize Core Data" {
        # "Do not delete, rename, or modify this frame.\n(this is used to determine panel behavior on exit)"
        # "originally closed?"
        # "exe?"
        # "If panel starts closed or is an EXE, then close it when we exit"
        n99 = property class="VI"() -> ("FP.State"=w231:T2)  [unwired: 2 in, 2 out]
        n100 = property class="App"() -> ("App.Kind"=w237:T3)  [unwired: 2 in, 2 out]
        n101 = control-ref of="Current VI Reference"() -> (w232:refnum<vi>)
        n102 = Equal?(x=w231, y=T2."Closed" ("Front Panel Window:State")) -> (x = y?=w229:bool)
        n103 = Equal?(x=w237, y=T3."Run Time System" ("Application:Kind")) -> (x = y?=w235:bool)
        n104 = Or(x=w229, y=w235) -> (x .or. y?=w233:bool)
        n105 = Bundle By Name(cluster=w234, "Core.Current VI Reference"=w232, "Core.Close Panel on Exit?"=w233) -> (w239:T6)
        n106 = call <vilib>:"Add State(s) to Queue__jki_lib_state_machine.vi"("State(s) in (\"\")"=w241) -> ("States Out"=w240:string)  [unwired: 14 in]
      }
      frame "Error Handler" {
        # "When running as sourcecode, this function will add previous state data to the error message to aid the developer in troubleshoot errors.\nIf run as an executable, no additional information is added to the error message."
        # "This state receives both Errors and Warnings which is how the Status of this wire can be FALSE"
        # "Unhandled Error -- Display it"
        # "Handle any errors or warnings here.\nYou can also output any states to clean-up after errors or warnings occur"
        # "Clear error or warning"
        n107 = disable-structure shown="Default" {
          disable-tunnel: w248 -> [w255 w256]
          disable-tunnel: w247 -> [w254 _]
          disable-tunnel: [w253 w256] -> w246
          frame condition #0 (active) {
            n108 = call <vilib>:"Append Error Details__jki_lib_state_machine.vi"("error in (no error)"=w255, "Previous State and Argument(s)"=w254) -> ("error out"=w253:errorcluster)  [unwired: 9 in]
          }
          frame condition #1 {
          }
        }
        n109 = call <vilib>:"General Error Handler.vi"("error in (no error)"=w246) -> ()  [unwired: 10 in, 5 out]
        n110 = call-poly <vilib>:"Select State(s)__jki_lib_state_machine.vi"("State(s) if True (\"\")"="/* Post Error States", "Select"=w246, "State(s) if False (\"\")"="/* Post Warning States") -> ("States Out"=w244:string)  [unwired: 12 in]
        n111 = call <vilib>:"Add State(s) to Queue__jki_lib_state_machine.vi"("State(s) in Front (\"\")"=w244, "State(s) in (\"\")"=w252) -> ("States Out"=w251:string)  [unwired: 13 in]
      }
      frame "Exit" {
        # "Do not put any code in this frame.\n(No errors that occur here will be handled.)"
        n112 = call <vilib>:"Add State(s) to Queue__jki_lib_state_machine.vi"("State(s) in (\"\")"=w262) -> ("States Out"=w261:string)  [unwired: 14 in]
      }
      frame "---------- Data ----------" {
        # "Do not put any code in this frame.\n(It is a separator no-op. You can make a copy of this frame to create a new Data frame)"
        n113 = call <vilib>:"Add State(s) to Queue__jki_lib_state_machine.vi"("State(s) in (\"\")"=w267) -> ("States Out"=w266:string)  [unwired: 14 in]
      }
      frame "Data: Initialize" {
        w268 = T5[] []  # issues
        w269 = T4 {"name"="", "sortable_name"="", "aliases"=[], "description"="", "site_detail_url"="", "count_of_issues"=0, "start_year"=0, "publisher_id"=0, "issue_ids"=[], "date_last_updated"=timestamp(0 s since 1904-01-01), "volume"=0, "cv_id"="", "volume type"=enum."Ongoing", "source_path"=path ""}  # volume
        w270 = map{string, i32} {}  # current volume map
        w271 = map{i32, map{string, i32}} {}  # vol  filter map
        w272 = TRUE  # Refresh all
        w273 = ""  # new volume
        w275 = i32[] []  # dup issues
        w276 = cluster{"cv_volumes":path, "cv_issues":path} {"cv_volumes"=path "D:/Comics/data/cv_volumes", "cv_issues"=path "D:/Comics/data/cv_issues"}  # root paths
        w278 = path[] []  # cv_vols
        w279 = T7 {"Current VI Reference"=refnum, "Close Panel on Exit?"=FALSE}  # Core
        # "Data names and types of shift register data are defined by this bundle."
        # "Initialize the shift-register data, here.\n(data names are defined by what you wire into the bundle function)"
        n114 = Bundle("Core"=w279, "cv_vols"=w278, "vol  filter map"=w271, "current volume map"=w270, "volume"=w269, "issues"=w268, "root paths"=w276, "dup issues"=w275, "manager_daemon"="manager_daemon", "new volume"=w273, "Refresh all"=w272) -> (w281:T6)  [unwired: 1 in]
        n115 = call <vilib>:"Add State(s) to Queue__jki_lib_state_machine.vi"("State(s) in (\"\")"=w283) -> ("States Out"=w282:string)  [unwired: 14 in]
      }
      frame "Data: Cleanup" {
        # "Cleanup any data and references, here.\n(this is called automatically, by the Macro: Exit)"
        n116 = Unbundle By Name(w285) -> ("Core.Current VI Reference"=w288:refnum<vi>)
        n117 = Close Reference(reference=w288, error in (no error)=w287) -> (error out=w286:errorcluster)
        n118 = call <vilib>:"Add State(s) to Queue__jki_lib_state_machine.vi"("State(s) in (\"\")"=w290) -> ("States Out"=w289:string)  [unwired: 14 in]
      }
      frame "---------- Events ----------" {
        n119 = call <vilib>:"Add State(s) to Queue__jki_lib_state_machine.vi"("State(s) in (\"\")"=w295) -> ("States Out"=w294:string)  [unwired: 14 in]
      }
      frame "Events: Register" {
        w305 = cluster{"My Event Data":bool} {"My Event Data"=FALSE}  # My User Event
        n120 = Unbundle By Name(w299) -> ("manager_daemon"=w298:refnum<class "manager_daemon.lvclass">)
        n121 = call "events.get.vi"("manager_daemon in"=w298) -> ("display volume event"=w296:refnum<user-event>, "refresh volume event"=w297:refnum<user-event>)  [unwired: 8 in, 1 out]
        n122 = property on="volume description" class="WebView2 Control (strict)"() -> ("Events"=w300:T8)  [unwired: 2 in, 2 out]
        n123 = Create User Event(user event datatype=w305, error in=w303) -> (user event=w306:refnum<user-event>, error out=w302:errorcluster)
        n124 = register-events(error in=w302, w306, w300, w297, w296) -> (reference out=w304:refnum<event-registration>, error out=w301:errorcluster)  [unwired: 1 in]
        n125 = call <vilib>:"Add State(s) to Queue__jki_lib_state_machine.vi"("State(s) in (\"\")"=w308) -> ("States Out"=w307:string)  [unwired: 14 in]
      }
      frame "Events: Unregister" {
        n126 = Unregister For Events(event registration refnum=w311, error in=w310) -> (error out=w309:errorcluster)
        n127 = call <vilib>:"Add State(s) to Queue__jki_lib_state_machine.vi"("State(s) in (\"\")"=w314) -> ("States Out"=w313:string)  [unwired: 14 in]
      }
      frame "---------- UI ----------" {
        n128 = call <vilib>:"Add State(s) to Queue__jki_lib_state_machine.vi"("State(s) in (\"\")"=w319) -> ("States Out"=w318:string)  [unwired: 14 in]
      }
      frame "UI: Display Volumes" {
        n129 = Unbundle By Name(w330) -> ("vol  filter map"=w332:map{i32, map{string, i32}})
        n130 = local read "Folder"() -> (w331:i32)
        n131 = Look In Map(map=w332, key=w331) -> (value=w328:map{string, i32})  [unwired: 1 in, 1 out]
        n132 = local read "target volume"() -> (w320:string)
        n133 = for {
          tunnel: w328 -> [w355] mode=indexing
          tunnel: [w354] -> w327 mode=indexing
          n134 = Unbundle By Name(w355) -> ("name"=w354:string)
        }
        n135 = local read "volumes"() -> (w323:i32)
        n136 = Empty String/Path?(string/path=w320) -> (empty?=w321:bool)
        n137 = case shown="False" w321 {
          tunnel: w327 -> [w340 w345]
          tunnel: w326 -> [w335 w344]
          tunnel: [w336 w343] -> w325
          tunnel: w323 -> [_ w342]
          tunnel: w322 -> [_ w341]
          tunnel: w320 -> [w339 _]
          frame False {
            n138 = Search 1D Array(1D array=w340, element=w339) -> (index of element=w337:i32)  [unwired: 1 in]
            n139 = local write "target volume"("") -> ()
            n140 = property on="volumes" class="LstBox (strict)"(error in=w335, "Item Names"=w340, "Val(Sgnl)"=w337) -> (error out=w336:errorcluster)  [unwired: 1 in, 1 out]
          }
          frame True {
            n141 = case shown="\"TRUE\"" w341 {
              tunnel: w345 -> [w349 w353]
              tunnel: w344 -> [w348 w352]
              tunnel: [w347 w351] -> w343
              tunnel: w342 -> [_ w350]
              frame "TRUE" {
                w346 = 0 ("Value (Signaling)")
                n142 = property on="volumes" class="LstBox (strict)"(error in=w348, "Item Names"=w349, "Val(Sgnl)"=w346, "Top Row"=w346) -> (error out=w347:errorcluster)  [unwired: 1 in, 1 out]
              }
              frame Default {
                n143 = property on="volumes" class="LstBox (strict)"(error in=w352, "Item Names"=w353, "Val(Sgnl)"=w350) -> (error out=w351:errorcluster)  [unwired: 1 in, 1 out]
              }
            }
          }
        }
        n144 = Bundle By Name(cluster=w330, "current volume map"=w328) -> (w329:T6)
        n145 = call <vilib>:"Add State(s) to Queue__jki_lib_state_machine.vi"("State(s) in (\"\")"=w334) -> ("States Out"=w333:string)  [unwired: 14 in]
      }
      frame "UI: Display Issues" {
        n146 = Unbundle By Name(w359) -> ("issues"=w358:T5[])
        n147 = Empty Array?(array=w358) -> (empty?=w357:bool)
        n148 = case shown="False" w357 {
          tunnel: w361 -> [w368 w380]
          tunnel: [w367 w380] -> w360
          tunnel: w358 -> [w366 _]
          tunnel: w356 -> [w365 _]
          frame False {
            n149 = for {
              tunnel: w366 -> [w379] mode=indexing
              tunnel: [w378] -> w369 mode=indexing
              n150 = Unbundle By Name(w379) -> ("sortable_name"=w378:string)
            }
            n151 = case shown="\"TRUE\"" w365 {
              tunnel: w369 -> [w373 w377]
              tunnel: w368 -> [w372 w376]
              tunnel: [w371 w375] -> w367
              frame Default {
                n152 = local read "issues"() -> (w370:i32)
                n153 = property on="issues" class="LstBox (strict)"(error in=w372, "Item Names"=w373, "Val(Sgnl)"=w370) -> (error out=w371:errorcluster)  [unwired: 1 in, 1 out]
              }
              frame "TRUE" {
                w374 = 0 ("Value (Signaling)")
                n154 = property on="issues" class="LstBox (strict)"(error in=w376, "Item Names"=w377, "Val(Sgnl)"=w374, "Top Row"=w374) -> (error out=w375:errorcluster)  [unwired: 1 in, 1 out]
              }
            }
          }
          frame True {
          }
        }
        n155 = call <vilib>:"Add State(s) to Queue__jki_lib_state_machine.vi"("State(s) in (\"\")"=w364) -> ("States Out"=w363:string)  [unwired: 14 in]
      }
      frame "UI: Ready" {
        n156 = call <vilib>:"Add State(s) to Queue__jki_lib_state_machine.vi"("State(s) in (\"\")"=w385) -> ("States Out"=w384:string)  [unwired: 14 in]
      }
      frame "UI: Populate Volume Info" {
        n157 = Unbundle By Name(w396) -> ("volume.date_last_updated"=w391:timestamp, "volume"=w387:T4, "volume.start_year"=→"Start Year":i32, "volume.count_of_issues"=→"issue count":i32, "volume.sortable_name"=→"Sortable Title":string, "volume.name"=w386:string, "volume.description"=w392:string, "volume.volume type"=w389:T1, "volume.site_detail_url"=→"URL":string)
        n158 = Format Date/Time String(seconds (now)=w391) -> (date/time string=→"last updated":string)  [unwired: 2 in]
        n159 = local write "Volume"(w387) -> ()
        n160 = local write "Title"(w386) -> ()
        n161 = local write "volume type"(w389) -> ()
        n162 = property on="volume description" class="WebView2 Control (strict)"(error in=w399, "Document Source"=w392) -> (error out=w398:errorcluster)  [unwired: 1 in, 1 out]
        n163 = call <vilib>:"Add State(s) to Queue__jki_lib_state_machine.vi"("State(s) in (\"\")"=w401) -> ("States Out"=w400:string)  [unwired: 14 in]
      }
      frame "UI: Populate Issue Info" {
        n164 = Unbundle By Name(w427) -> ("issues"=w426:T5[])
        n165 = local read "issues"() -> (w425:i32)
        n166 = Index Array(array=w426, index=w425) -> (element=w424:T5)
        n167 = Unbundle By Name(w424) -> ("store_date"=→"Rel Date":timestamp, "cover_date"=w403:timestamp, "id"=→"Issue ID":i32, "name"=→"Issue Title":string, "issue_number"=→"Issue Number":string, "cover_url"=w420:string, "description"=w415:string, "characters"=w414, "concepts"=w412, "storyArcs"=w410, "teams"=w408, "creators"=w406)
        n168 = property on="issue description" class="WebView2 Control (strict)"(error in=w419, "Document Source"=w415) -> (error out=w418:errorcluster)  [unwired: 1 in, 1 out]
        n169 = property on="issue cover" class="WebView2 Control (strict)"(error in=w419, "URL"=w420) -> (error out=w417:errorcluster)  [unwired: 1 in, 1 out]
        n170 = local write "Cover Date"(w403) -> ()
        n171 = for {
          tunnel: w414 -> [w443]
          tunnel: [w442] -> w413 mode=indexing
          n172 = Unbundle By Name(w443) -> ("name"=w442)
        }
        "Characters" <- w413
        n173 = for {
          tunnel: w412 -> [w441]
          tunnel: [w440] -> w411 mode=indexing
          n174 = Unbundle By Name(w441) -> ("name"=w440)
        }
        "Concepts" <- w411
        n175 = for {
          tunnel: w410 -> [w439]
          tunnel: [w438] -> w409 mode=indexing
          n176 = Unbundle By Name(w439) -> ("name"=w438)
        }
        "StoryArcs" <- w409
        n177 = for {
          tunnel: w408 -> [w437]
          tunnel: [w436] -> w407 mode=indexing
          n178 = Unbundle By Name(w437) -> ("name"=w436)
        }
        "Teams" <- w407
        n179 = Merge Errors(w417, w418) -> (w416:errorcluster)
        n180 = for {
          tunnel: w406 -> [w435]
          tunnel: [w432] -> w405 mode=indexing
          tunnel: " - " ("string") -> [w431]
          n181 = Unbundle By Name(w435) -> ("name"=w434, "role"=w433)
          n182 = Concatenate Strings(w434, w431, w433) -> (w432:string)
        }
        "Creators" <- w405
        n183 = call <vilib>:"Add State(s) to Queue__jki_lib_state_machine.vi"("State(s) in (\"\")"=w430) -> ("States Out"=w429:string)  [unwired: 14 in]
      }
      frame "UI: Initialize" {
        # "Initialize the User Interface, here.\n(this is called automatically, by the Macro: Initialize)"
        n184 = call <vilib>:"Add State(s) to Queue__jki_lib_state_machine.vi"("State(s) in Front (\"\")"="Actions: Populate cv_vols\nActions: create volume filter map\nUI: Display Volumes >> TRUE\nActions: Load Volume\nUI: Ready" ("State(s) in Front (\"\")"), "State(s) in (\"\")"=w449) -> ("States Out"=w448:string)  [unwired: 13 in]
      }
      frame "UI: Uninitialize" {
        # "Cleanup the User Interface, here.\n(this is called automatically, by the Macro: Exit)"
        n185 = call <vilib>:"Add State(s) to Queue__jki_lib_state_machine.vi"("State(s) in (\"\")"=w454) -> ("States Out"=w453:string)  [unwired: 14 in]
      }
      frame "UI: Cursor Set" {
        # "Argument"
        # "Set and Unset Cursor Busy.\n(Usage: \"UI: Cursor Set >> Busy|Idle\")"
        n186 = case shown="\"Idle\", Default" w456 {
          tunnel: w458 -> [w463 w465]
          tunnel: [w462 w464] -> w457
          frame "Idle", Default {
            n187 = call <vilib>:"Unset Busy.vi"("error in (no error)"=w463) -> ("error out"=w462:errorcluster)  [unwired: 10 in]
          }
          frame "Busy" {
            n188 = call <vilib>:"Set Busy.vi"("error in (no error)"=w465) -> ("error out"=w464:errorcluster)  [unwired: 9 in, 1 out]
          }
        }
        n189 = call <vilib>:"Add State(s) to Queue__jki_lib_state_machine.vi"("State(s) in (\"\")"=w461) -> ("States Out"=w460:string)  [unwired: 14 in]
      }
      frame "UI: Front Panel State" {
        # "Argument"
        # "Set Front Panel Open or Closed\n(Usage: \"UI: Front Panel State >> Open|Close\")"
        n190 = Unbundle By Name(w469) -> ("Core.Current VI Reference"=w468:refnum<vi>)
        n191 = case shown="\"Open\", \"Standard\", Default" w467 {
          tunnel: w471 -> [w479 w494 w505 w518 w531]
          tunnel: [w481 w495 w507 w520 w533] -> w470
          tunnel: w468 -> [w480 w492 w506 w519 w532]
          frame "Open", "Standard", Default {
            w474 = T2."Standard" ("State")
            n192 = property class="VI"(reference=w480, error in=w479) -> (reference out=w477:refnum<vi>, error out=w478:errorcluster, "FP.State"=w476:T2)
            n193 = Not Equal?(x=w476, y=w474) -> (x != y?=w475:bool)
            n194 = case shown="False" w475 {
              tunnel: [w485 w487] -> w481
              tunnel: w478 -> [w484 w487]
              tunnel: w477 -> [w483 _]
              tunnel: w474 -> [w482 _]
              frame True {
                n195 = invoke class="VI" method="FP.Open"(reference=w483, error in=w484, "Activate"=TRUE, "State"=w482) -> (error out=w485:errorcluster)  [unwired: 1 in, 4 out]
              }
              frame False {
              }
            }
          }
          frame "Close", "Closed" {
            n196 = property class="VI"(reference=w492, error in=w494) -> (reference out=w491:refnum<vi>, error out=w493:errorcluster, "FP.State"=w489:T2)
            n197 = Not Equal?(x=w489, y=T2."Closed" ("Front Panel Window:State")) -> (x != y?=w488:bool)
            n198 = case shown="True" w488 {
              tunnel: [w496 w499] -> w495
              tunnel: w493 -> [w496 w498]
              tunnel: w491 -> [_ w497]
              frame False {
              }
              frame True {
                n199 = invoke class="VI" method="FP.Close"(reference=w497, error in=w498) -> (error out=w499:errorcluster)  [unwired: 1 in, 2 out]
              }
            }
          }
          frame "Hidden", "Hide" {
            w500 = T2."Hidden" ("State")
            n200 = property class="VI"(reference=w506, error in=w505) -> (reference out=w503:refnum<vi>, error out=w504:errorcluster, "FP.State"=w502:T2)
            n201 = Not Equal?(x=w502, y=w500) -> (x != y?=w501:bool)
            n202 = case shown="True" w501 {
              tunnel: [w511 w512] -> w507
              tunnel: w504 -> [w510 w512]
              tunnel: w503 -> [w509 _]
              tunnel: w500 -> [w508 _]
              frame True {
                n203 = invoke class="VI" method="FP.Open"(reference=w509, error in=w510, "State"=w508) -> (error out=w511:errorcluster)  [unwired: 2 in, 4 out]
              }
              frame False {
              }
            }
          }
          frame "Minimize", "Minimized" {
            w513 = T2."Minimized" ("State")
            n204 = property class="VI"(reference=w519, error in=w518) -> (reference out=w516:refnum<vi>, error out=w517:errorcluster, "FP.State"=w515:T2)
            n205 = Not Equal?(x=w515, y=w513) -> (x != y?=w514:bool)
            n206 = case shown="True" w514 {
              tunnel: [w524 w525] -> w520
              tunnel: w517 -> [w523 w525]
              tunnel: w516 -> [w522 _]
              tunnel: w513 -> [w521 _]
              frame True {
                n207 = invoke class="VI" method="FP.Open"(reference=w522, error in=w523, "State"=w521) -> (error out=w524:errorcluster)  [unwired: 2 in, 4 out]
              }
              frame False {
              }
            }
          }
          frame "Maximize", "Maximized" {
            w526 = T2."Maximized" ("State")
            n208 = property class="VI"(reference=w532, error in=w531) -> (reference out=w529:refnum<vi>, error out=w530:errorcluster, "FP.State"=w528:T2)
            n209 = Not Equal?(x=w528, y=w526) -> (x != y?=w527:bool)
            n210 = case shown="True" w527 {
              tunnel: [w537 w538] -> w533
              tunnel: w530 -> [w536 w538]
              tunnel: w529 -> [w535 _]
              tunnel: w526 -> [w534 _]
              frame True {
                n211 = invoke class="VI" method="FP.Open"(reference=w535, error in=w536, "State"=w534) -> (error out=w537:errorcluster)  [unwired: 2 in, 4 out]
              }
              frame False {
              }
            }
          }
        }
        n212 = call <vilib>:"Add State(s) to Queue__jki_lib_state_machine.vi"("State(s) in (\"\")"=w473) -> ("States Out"=w472:string)  [unwired: 14 in]
      }
      frame "---------- Macro ----------" {
        # "Do not put any code in this frame.\n(It is a separator no-op. You can make a copy of this frame to create a new Macro frame)"
        n213 = call <vilib>:"Add State(s) to Queue__jki_lib_state_machine.vi"("State(s) in (\"\")"=w543) -> ("States Out"=w542:string)  [unwired: 14 in]
      }
      frame "Macro: Initialize" {
        # "Initialization Macro\n(This is called once, when the VI starts)"
        n214 = call <vilib>:"Add State(s) to Queue__jki_lib_state_machine.vi"("State(s) in Front (\"\")"="Data: Initialize\nInitialize Core Data\nEvents: Register\nUI: Initialize\nUI: Front Panel State >> Open", "State(s) in (\"\")"=w549) -> ("States Out"=w548:string)  [unwired: 13 in]
      }
      frame "Macro: Exit" {
        # "Exit Macro\n(This is called once, when the VI exits)"
        n215 = Unbundle By Name(w557) -> ("Core.Close Panel on Exit?"=w552:bool)
        n216 = call <vilib>:"Conditional State String__jki_lib_state_machine.vi"("Do State(s)?"=w552, "State"="UI: Front Panel State >> Close") -> ("State Out"=w551:string)  [unwired: 7 in]
        n217 = call <vilib>:"Add State(s) to Queue__jki_lib_state_machine.vi"("State(s) in (\"\")"=w551, "State(s) at Back (\"\")"="UI: Uninitialize\nData: Cleanup\nEvents: Unregister\nExit") -> ("States Out"=w555:string)  [unwired: 13 in]
        n218 = call <vilib>:"Add State(s) to Queue__jki_lib_state_machine.vi"("State(s) in Front (\"\")"=w555, "State(s) in (\"\")"=w559) -> ("States Out"=w558:string)  [unwired: 13 in]
      }
      frame "---------- Actions ----------" {
        n219 = call <vilib>:"Add State(s) to Queue__jki_lib_state_machine.vi"("State(s) in (\"\")"=w564) -> ("States Out"=w563:string)  [unwired: 14 in]
      }
      frame "Actions: Delete Issue" {
        n220 = Unbundle By Name(w583) -> ("current volume map"=w567:map{string, i32}, "manager_daemon"=w580:refnum<class "manager_daemon.lvclass">, "volume.issue_ids"=w582:i32[])
        n221 = property on="volumes" class="LstBox (strict)"() -> ("Item Names"=w568:string[], "Value"=w569:i32)  [unwired: 2 in, 2 out]
        n222 = local read "issues"() -> (w581:i32)
        n223 = Index Array(array=w568, index=w569) -> (element=w566:string)
        n224 = Index Array(array=w582, index=w581) -> (element=w578:i32)
        n225 = Look In Map(map=w567, key=w566) -> (value=w565:i32)  [unwired: 1 in, 1 out]
        n226 = Build Array(w578) -> (w577:i32[])
        n227 = call "delete issues.vi"("error in (no error)"=w579, "issue path"=w577, "manager_daemon in"=w580) -> ("error out"=w575:errorcluster, "manager_daemon out"=w576:refnum<class "manager_daemon.lvclass">)  [unwired: 7 in]
        n228 = call "volume.get.vi"("error in (no error)"=w575, "volume ID"=w565, "manager_daemon in"=w576) -> ("error out"=w574:errorcluster, "volume"=w571:T4, "manager_daemon out"=w572:refnum<class "manager_daemon.lvclass">)  [unwired: 6 in]
        n229 = call "issues.get.vi"("error in (no error)"=w574, "volume ID"=w565, "manager_daemon in"=w572) -> ("error out"=w573:errorcluster, "issues"=w570:T5[])  [unwired: 6 in, 1 out]
        n230 = Bundle By Name(cluster=w583, "volume"=w571, "issues"=w570) -> (w584:T6)
        n231 = call <vilib>:"Add State(s) to Queue__jki_lib_state_machine.vi"("State(s) in (\"\")"=w587) -> ("States Out"=w586:string)  [unwired: 14 in]
      }
      frame "Actions: Select New Volume" {
        n232 = Unbundle By Name(w594) -> ("current volume map"=w593:map{string, i32}, "new volume"=w591:string)
        n233 = for {
          tunnel: w593 -> [w599] mode=indexing
          tunnel: [w598] -> w592 mode=indexing
          n234 = Unbundle By Name(w599) -> ("name"=w598:string)
        }
        n235 = Search 1D Array(1D array=w592, element=w591) -> (index of element=w590:i32)  [unwired: 1 in]
        n236 = property on="volumes" class="LstBox (strict)"(error in=w589, "Val(Sgnl)"=w590) -> (error out=w588:errorcluster)  [unwired: 1 in, 1 out]
        n237 = call <vilib>:"Add State(s) to Queue__jki_lib_state_machine.vi"("State(s) in (\"\")"=w597) -> ("States Out"=w596:string)  [unwired: 14 in]
      }
      frame "Actions: Change Title" {
        n238 = Unbundle By Name(w622) -> ("volume"=w623:T4, "volume.start_year"=w607:i32)
        n239 = local read "Title"() -> (w611:string)
        n240 = Unbundle By Name(w622) -> ("manager_daemon"=w603:refnum<class "manager_daemon.lvclass">, "root paths.cv_volumes"=w616:path, "current volume map"=w621:map{string, i32})
        n241 = local read "volumes"() -> (w620:i32)
        n242 = call "MakeSortable.vi"("string in"=w611) -> ("string out"=w610:string)
        n243 = call "remove.invalid.chars.vi"("string in"=w610) -> ("string out"=w608:string)
        n244 = Index Array(array=w621, index=w620) -> (element=w619)
        n245 = Format Into String(format string="%s (%d)", w608, w607) -> (resulting string=w606:string)  [unwired: 2 in, 1 out]
        n246 = Unbundle By Name(w619) -> ("path"=w618)
        n247 = Delete(path (use dialog)=w618, error in=w617) -> (error out=w615:errorcluster)  [unwired: 3 in, 2 out]
        n248 = Bundle By Name(cluster=w623, "name"=w611, "sortable_name"=w606) -> (w612:T4)
        n249 = call "create.volume.filename.vi"("volume"=w612) -> ("json filename"=w600:string)  [unwired: 10 in]
        n250 = call <vilib>:"Flatten To JSON String.vi"("error in"=w615, "Variant"=w612) -> ("error out"=w614:errorcluster, "JSON String"=w613:string)  [unwired: 8 in]
        n251 = call-poly <userlib>:"Strip Path Extension__ogtk.vi"("path"=w600) -> ("root"=w601:string)  [unwired: 1 out]
        n252 = Build Path(base path=w616, name or relative path=w600) -> (appended path=w602:path)
        n253 = Bundle By Name(cluster=w622, "volume"=w612, "new volume"=w601) -> (w624:T6)
        n254 = Write to Text File(file (use dialog)=w602, text=w613, error in=w614) -> (error out=w605:errorcluster)  [unwired: 1 in, 2 out]
        n255 = call "update volume.vi"("error in (no error)"=w605, "volume data"=w602, "manager_daemon in"=w603) -> ("error out"=w604:errorcluster)  [unwired: 7 in, 1 out]
        n256 = call <vilib>:"Add State(s) to Queue__jki_lib_state_machine.vi"("State(s) in (\"\")"=w627) -> ("States Out"=w626:string)  [unwired: 14 in]
      }
      frame "Actions: Change Dates to Rel Date" {
        n257 = Unbundle By Name(w635) -> ("issues"=w637:T5[], "root paths.cv_issues"=w636:path, "manager_daemon"=w628:refnum<class "manager_daemon.lvclass">)
        n258 = for {
          tunnel: w637 -> [w651] mode=indexing
          tunnel: w636 -> [w647]
          tunnel: [w646] -> w634 mode=indexing
          shift-right: [w642] -> w631
          shift-left: w632 -> [w643]
          tunnel: [w641] -> w629 mode=indexing
          n259 = in-place {
            in-place-border: [w652] -> w649
            n260 = in-place-cluster #2(w651) -> ("store_date"=w653:timestamp, "id"=w652:i32)  [unwired: 1 out]
            n261 = in-place-cluster #2("cover_date"=w653, "store_date"=w653, "id"=w652) -> (w646:T5)
          }
          n262 = Format Into String(format string="%d.json", w649) -> (resulting string=w648:string)  [unwired: 2 in, 1 out]
          n263 = Build Path(base path=w647, name or relative path=w648) -> (appended path=w641:path)
          n264 = call <vilib>:"Flatten To JSON String.vi"("error in"=w643, "Variant"=w646) -> ("error out"=w644:errorcluster, "JSON String"=w645:string)  [unwired: 8 in]
          n265 = Write to Text File(file (use dialog)=w641, text=w645, error in=w644) -> (error out=w642:errorcluster)  [unwired: 1 in, 2 out]
        }
        n266 = Bundle By Name(cluster=w635, "issues"=w634) -> (w633:T6)
        n267 = call "update issues.vi"("error in (no error)"=w631, "Volume Path"=w629, "manager_daemon in"=w628) -> ("error out"=w630:errorcluster)  [unwired: 7 in, 1 out]
        n268 = call <vilib>:"Add State(s) to Queue__jki_lib_state_machine.vi"("State(s) in (\"\")"=w640) -> ("States Out"=w639:string)  [unwired: 14 in]
      }
      frame "Actions: Draw Issues" {
        n269 = Unbundle By Name(w662) -> ("volume.volume type"=w654:T1, "volume.sortable_name"=w655:string, "issues"=w661:T5[])
        n270 = for {
          tunnel: w661 -> [w668] mode=indexing
          tunnel: [w667] -> w659 mode=indexing
          tunnel: [w666] -> w658 mode=indexing
          n271 = Unbundle By Name(w668) -> ("issue_number"=w666:string, "cover_date"=w667:timestamp)
        }
        n272 = control-ref of="issue chart"() -> (w660:refnum<vi>)
        n273 = call "plot.issues.vi"("volume.volume type"=w654, "volume_name"=w655, "error in (no error)"=w657, "cover_dates"=w659, "issue_numbers"=w658, "picture ref"=w660) -> ("error out"=w656:errorcluster)  [unwired: 4 in, 1 out]
        n274 = call <vilib>:"Add State(s) to Queue__jki_lib_state_machine.vi"("State(s) in (\"\")"=w665) -> ("States Out"=w664:string)  [unwired: 14 in]
      }
      frame "Actions: Clean Cover Dates" {
        n275 = Unbundle By Name(w677) -> ("manager_daemon"=w669:refnum<class "manager_daemon.lvclass">, "issues"=w679:T5[], "dup issues"=w678:i32[], "root paths.cv_issues"=w674:path)
        n276 = call "interpolate.issue.dates.vi"("dup issues"=w678, "issues"=w679) -> ("issues out"=w675:T9[])  [unwired: 9 in]
        n277 = for {
          tunnel: w678 -> [w693] mode=indexing
          tunnel: w675 -> [w694]
          tunnel: w674 -> [w688]
          shift-right: [w684] -> w672
          shift-left: w673 -> [w685]
          tunnel: [w683] -> w670 mode=indexing
          n278 = Index Array(array=w694, index=w693) -> (element=w692:T9)
          n279 = Unbundle By Name(w692) -> ("id"=w691:i32)
          n280 = call <vilib>:"Flatten To JSON String.vi"("error in"=w685, "Variant"=w692) -> ("error out"=w686:errorcluster, "JSON String"=w687:string)  [unwired: 8 in]
          n281 = Format Into String(format string="%d.json", w691) -> (resulting string=w689:string)  [unwired: 2 in, 1 out]
          n282 = Build Path(base path=w688, name or relative path=w689) -> (appended path=w683:path)
          n283 = Write to Text File(file (use dialog)=w683, text=w687, error in=w686) -> (error out=w684:errorcluster)  [unwired: 1 in, 2 out]
        }
        n284 = Bundle By Name(cluster=w677, "issues"=w675) -> (w676:T6)
        n285 = call "update issues.vi"("error in (no error)"=w672, "Volume Path"=w670, "manager_daemon in"=w669) -> ("error out"=w671:errorcluster)  [unwired: 7 in, 1 out]
        n286 = call <vilib>:"Add State(s) to Queue__jki_lib_state_machine.vi"("State(s) in (\"\")"=w682) -> ("States Out"=w681:string)  [unwired: 14 in]
      }
      frame "Actions: Delete Volume" {
        n287 = Unbundle By Name(w709) -> ("manager_daemon"=w700:refnum<class "manager_daemon.lvclass">, "root paths.cv_issues"=w705:path, "volume.issue_ids"=w706:i32[], "current volume map"=w708:map{string, i32})
        n288 = local read "volumes"() -> (w707:i32)
        n289 = Index Array(array=w708, index=w707) -> (element=w704)
        n290 = Unbundle By Name(w704) -> ("path"=w699)
        n291 = Delete(path (use dialog)=w699, error in=w703) -> (error out=w702:errorcluster)  [unwired: 3 in, 2 out]
        n292 = call "delete volume.vi"("error in (no error)"=w702, "issue path"=w699, "manager_daemon in"=w700) -> ("error out"=w701:errorcluster, "manager_daemon out"=w696:refnum<class "manager_daemon.lvclass">)  [unwired: 7 in]
        n293 = for {
          tunnel: w706 -> [w719] mode=indexing
          tunnel: w705 -> [w717]
          shift-right: [w716] -> w698
          shift-left: w701 -> [w714]
          tunnel: [w713] -> w695 mode=indexing
          n294 = Format Into String(format string="%d.json", w719) -> (resulting string=w718:string)  [unwired: 2 in, 1 out]
          n295 = Build Path(base path=w717, name or relative path=w718) -> (appended path=w715:path)
          n296 = Delete(path (use dialog)=w715, error in=w714) -> (deleted path=w713:path, error out=w716:errorcluster)  [unwired: 3 in, 1 out]
        }
        n297 = call "delete issues.vi"("error in (no error)"=w698, "issue path"=w695, "manager_daemon in"=w696) -> ("error out"=w697:errorcluster)  [unwired: 7 in, 1 out]
        n298 = call <vilib>:"Add State(s) to Queue__jki_lib_state_machine.vi"("State(s) in (\"\")"=w712) -> ("States Out"=w711:string)  [unwired: 14 in]
      }
      frame "Actions: Sort Volume" {
        n299 = Unbundle By Name(w730) -> ("manager_daemon"=w722:refnum<class "manager_daemon.lvclass">, "current volume map"=w729:map{string, i32}, "root paths.cv_issues"=w728:path)
        n300 = local read "volumes"() -> (w726:i32)
        n301 = Index Array(array=w729, index=w726) -> (element=w725)
        n302 = Unbundle By Name(w725) -> ("path"=w721)
        n303 = call "sort.volume.issues.vi"("error in"=w731, "issues path"=w728, "volume path"=w721) -> ("error out"=w727:errorcluster)  [unwired: 8 in]
        n304 = property on="volumes" class="LstBox (strict)"(error in=w727, "Val(Sgnl)"=w726) -> (error out=w724:errorcluster)  [unwired: 1 in, 1 out]
        n305 = call "update volume.vi"("error in (no error)"=w724, "volume data"=w721, "manager_daemon in"=w722) -> ("error out"=w723:errorcluster)  [unwired: 7 in, 1 out]
        n306 = call <vilib>:"Add State(s) to Queue__jki_lib_state_machine.vi"("State(s) in (\"\")"=w734) -> ("States Out"=w733:string)  [unwired: 14 in]
      }
      frame "Actions: Update Volume Type" {
        n307 = Unbundle By Name(w744) -> ("manager_daemon"=w741:refnum<class "manager_daemon.lvclass">, "current volume map"=w739:map{string, i32}, "volume.sortable_name"=w735:string)
        n308 = local read "volume type"() -> (w743:T1)
        n309 = Bundle By Name(cluster=w744, "volume.volume type"=w743, "new volume"=w735) -> (w737:T6)
        n310 = Look In Map(map=w739, key=w735) -> (value=w740:i32)  [unwired: 1 in, 1 out]
        n311 = Unbundle By Name(w737) -> ("volume"=w736:T4)
        n312 = call "update volume.vi"("volume id"=w740, "error in (no error)"=w738, "volume data"=w736, "manager_daemon in"=w741) -> ("error out"=w742:errorcluster)  [unwired: 6 in, 1 out]
        n313 = call <vilib>:"Add State(s) to Queue__jki_lib_state_machine.vi"("State(s) in (\"\")"=w747) -> ("States Out"=w746:string)  [unwired: 14 in]
      }
      frame "Actions: Move Issue" {
        n314 = Unbundle By Name(w750) -> ("current volume map"=w754:map{string, i32}, "volume.sortable_name"=w748:string, "manager_daemon"=w757:refnum<class "manager_daemon.lvclass">, "volume"=w763:T4, "volume.issue_ids"=w768:i32[])
        n315 = local read "issues"() -> (w764:i32)
        n316 = case shown="\"up\"" w753 {
          tunnel: w764 -> [w774 w777 _]
          tunnel: [w773 w776 0] -> w759
          tunnel: w752 -> [w772 w775 w779]
          tunnel: [w772 w775 w778] -> w751
          frame "down", Default {
            n317 = Decrement(x=w774) -> (x-1=w773:i32)
          }
          frame "up" {
            n318 = Increment(x=w777) -> (x+1=w776:i32)
          }
          frame "top" {
            n319 = property on="issues" class="LstBox (strict)"(error in=w779, "Top Row"=0) -> (error out=w778:errorcluster)  [unwired: 1 in, 1 out]
          }
        }
        n320 = Delete From Array(array=w768, length=1, index=w764) -> (deleted portion=w765:i32[], array with subset deleted=w766:i32[])
        n321 = Look In Map(map=w754, key=w748) -> (value=w756:i32)  [unwired: 1 in, 1 out]
        n322 = Bundle By Name(cluster=w750, "new volume"=w748) -> (w749:T6)
        n323 = Insert Into Array(array=w766, index=w759, new element=w765) -> (w762:i32[])
        n324 = local write "issues"(w759) -> ()
        n325 = Bundle By Name(cluster=w763, "issue_ids"=w762) -> (w755:T4)
        n326 = call "update volume.vi"("volume id"=w756, "error in (no error)"=w751, "volume data"=w755, "manager_daemon in"=w757) -> ("error out"=w758:errorcluster)  [unwired: 6 in, 1 out]
        n327 = local read "volumes"() -> (w761:i32)
        n328 = property on="volumes" class="LstBox (strict)"(error in=w758, "Val(Sgnl)"=w761) -> (error out=w760:errorcluster)  [unwired: 1 in, 1 out]
        n329 = call <vilib>:"Add State(s) to Queue__jki_lib_state_machine.vi"("State(s) in (\"\")"=w771) -> ("States Out"=w770:string)  [unwired: 14 in]
      }
      frame "Actions: Change Volume" {
        n330 = Unbundle By Name(w786) -> ("current volume map"=w787:map{string, i32}, "volume.sortable_name"=w784:string, "manager_daemon"=w790:refnum<class "manager_daemon.lvclass">, "volume"=w794:T4)
        n331 = Look In Map(map=w787, key=w784) -> (value=w789:i32)  [unwired: 1 in, 1 out]
        n332 = Bundle By Name(cluster=w786, "new volume"=w784) -> (w785:T6)
        n333 = local read "Volume"() -> (w782:i32)
        n334 = Bundle By Name(cluster=w794, "volume"=w782) -> (w788:T4)
        n335 = call "update volume.vi"("volume id"=w789, "error in (no error)"=w783, "volume data"=w788, "manager_daemon in"=w790) -> ("error out"=w791:errorcluster)  [unwired: 6 in, 1 out]
        n336 = local read "volumes"() -> (w793:i32)
        n337 = property on="volumes" class="LstBox (strict)"(error in=w791, "Val(Sgnl)"=w793) -> (error out=w792:errorcluster)  [unwired: 1 in, 1 out]
        n338 = call <vilib>:"Add State(s) to Queue__jki_lib_state_machine.vi"("State(s) in (\"\")"=w797) -> ("States Out"=w796:string)  [unwired: 14 in]
      }
      frame "Actions: Load Volume" {
        n339 = Unbundle By Name(w808) -> ("manager_daemon"=w802:refnum<class "manager_daemon.lvclass">, "current volume map"=w804:map{string, i32})
        n340 = property on="volumes" class="LstBox (strict)"() -> ("Item Names"=w806:string[], "Value"=w805:i32)  [unwired: 2 in, 2 out]
        n341 = Index Array(array=w806, index=w805) -> (element=w803:string)
        n342 = Look In Map(map=w804, key=w803) -> (value=w799:i32)  [unwired: 1 in, 1 out]
        n343 = call "volume.get.vi"("error in (no error)"=w801, "volume ID"=w799, "manager_daemon in"=w802) -> ("error out"=w800:errorcluster, "volume"=w798:T4)  [unwired: 6 in, 1 out]
        n344 = Bundle By Name(cluster=w808, "volume"=w798) -> (w807:T6)
        n345 = call <vilib>:"Add State(s) to Queue__jki_lib_state_machine.vi"("State(s) in (\"\")"=w811) -> ("States Out"=w810:string)  [unwired: 14 in]
      }
      frame "Actions: Load Issues" {
        n346 = Unbundle By Name(w828) -> ("manager_daemon"=w821:refnum<class "manager_daemon.lvclass">, "current volume map"=w820:map{string, i32})
        n347 = property on="volumes" class="LstBox (strict)"(error in=w816) -> (error out=w817:errorcluster, "Item Names"=w823:string[], "Value"=w822:i32)  [unwired: 1 in, 1 out]
        n348 = Index Array(array=w823, index=w822) -> (element=w819:string)
        n349 = Look In Map(map=w820, key=w819) -> (value=w818:i32)  [unwired: 1 in, 1 out]
        n350 = call "issues.get.vi"("error in (no error)"=w817, "volume ID"=w818, "manager_daemon in"=w821) -> ("error out"=w812:errorcluster, "issues"=w815:T5[])  [unwired: 6 in, 1 out]
        n351 = for {
          tunnel: w815 -> [w833] mode=indexing
          tunnel: [w832] -> w814 mode=indexing
          tunnel: [w831] -> w813 mode=indexing
          n352 = Unbundle By Name(w833) -> ("cover_date"=w832:timestamp, "issue_number"=w831:string)
        }
        n353 = call-poly <userlib>:"Remove Duplicates from 1D Array__ogtk.vi"("Input Array"=w814) -> ("indices of removed elements"=w825:i32[])  [unwired: 1 out]
        n354 = Empty Array?(array=w825) -> (empty?=→"Unique Dates":bool)
        n355 = for {
          tunnel: w813 -> [w835]
          tunnel: w825 -> [w836] mode=indexing
          tunnel: [w834] -> w824 mode=indexing
          n356 = Index Array(array=w835, index=w836) -> (element=w834:string)
        }
        "dup issue dates" <- w824
        n357 = Bundle By Name(cluster=w828, "dup issues"=w825, "issues"=w815) -> (w827:T6)
      }
      frame "Actions: Populate cv_vols" {
        n358 = Unbundle By Name(w838) -> ("root paths.cv_volumes"=w837:path)
        n359 = call <vilib>:"Recursive File List.vi"("pattern"="*.json", "error in (no error)"=w840, "Folder Path"=w837) -> ("error out"=w841:errorcluster, "All Files in Dir"=w843:path[])  [unwired: 4 in, 3 out]
        n360 = Bundle By Name(cluster=w838, "cv_vols"=w843) -> (w842:T6)
        n361 = call <vilib>:"Add State(s) to Queue__jki_lib_state_machine.vi"("State(s) in (\"\")"=w846) -> ("States Out"=w845:string)  [unwired: 14 in]
      }
      frame "Actions: create volume filter map" {
        n362 = Unbundle By Name(w850) -> ("manager_daemon"=w849:refnum<class "manager_daemon.lvclass">)
        n363 = call "folder.volume.map.get.vi"("error in (no error)"=w852, "manager_daemon in"=w849) -> ("error out"=w848:errorcluster, "vol_ map"=w847:map{i32, map{string, i32}})  [unwired: 7 in, 1 out]
        n364 = Bundle By Name(cluster=w850, "vol  filter map"=w847) -> (w853:T6)
      }
    }
  }
